vi "main.vi"(8 "error in (no error)":errorcluster, 10 "stages":refnum<class "_stage.lvclass">[](array[class]), 11 "_camera":refnum<class "_camera.lvclass">) -> ()   [LabVIEW 2019]
uses:
  _camera/_camera.lvlibp/_cameraClass/_camera.lvclass
  _stage/_stage.lvlibp/_stageClass/_stage.lvclass
  _dataProcessing/_dataProcessing.lvlibp/_dataProcessingClass/_dataProcessing.lvclass
  <vilib>/Analysis/6fits.llb/Curve Fitting Criteria.ctl
  data_process.ctl
  state.ctl
  <vilib>/Analysis/baseanly.llb/Mean (DBL).vi
  _camera/_camera.lvlibp/_cameraClass/Write stage positions.vi
  _camera/_camera.lvlibp/_cameraClass/Read camera name and version.vi
  _camera/_camera.lvlibp/_cameraClass/Read wavelength.vi
  _camera/_camera.lvlibp/_cameraClass/Write background.vi
  <vilib>/gmath/NumericalOptimization/Nonlinear Curve Fit LM formula string.vi
  _camera/_camera.lvlibp/_cameraClass/Write wavelength.vi
  <vilib>/Utility/file.llb/Read Delimited Spreadsheet (DBL).vi
  <vilib>/Utility/config.llb/Write Key (Double).vi
  <vilib>/Utility/config.llb/Write Key (String).vi
  <vilib>/Utility/config.llb/Read Key (Double).vi
  <vilib>/Utility/config.llb/Read Key (String).vi
  <vilib>/Analysis/NI_AALBase.lvlib
  <vilib>/Utility/Data Type/NI_Data Type.lvlib
  <vilib>/Analysis/NI_AALPro.lvlib
  <vilib>/Utility/config.llb/NI_LVConfig.lvlib
  <vilib>/gmath/NI_Gmath.lvlib
panel:
  in  "is stage reversed?":bool=TRUE
  in  "Experimenter":string="who are you?"
  in  "Title":string="A clever title"
  in  "Experimental parameters (will be saved)":string="sample:\nsolvent:\ncuvette:\noptical density:\nexcitation wavelength:\nexcitation power:\nexcitation spot size:\nexcitation fluence: \nprobe spot size:\ncomment:"
  in  "method":T1 items=["Least Square", "Least Absolute Residual", "Bisquare"]
  out "amplitude":dbl format="%#_3g"
  out "power":dbl format="%#_3g"
  out "offset":dbl format="%#_3g"
  in  "parameter bounds":T2={"amp min"=-inf, "amp max"=inf, "power min"=-inf, "power max"=inf, "offset min"=0.0, "offset max"=600.0}
  out "current scan":i32
  in  "N scans":u16=5
  in  "sample":string="testSample"
  in  "Experiment":string="testExp"
  in  "center cursor":bool=TRUE
  in  "save flag":bool
  in  "save type":bool[](array[boolean])=[FALSE, FALSE, FALSE, FALSE]
  in  "data folder":path=path "Z:/11 Setups/04 NOPA TA/01 Data"
  out "progress":u8(slide) scale=0.0..100.0
  out "scan progress":u8(slide) scale=0.0..100.0
  out "Cursor position (wl)":dbl[](array[numeric])
  out "Cursor position (idx)":dbl[](array[numeric])
  in  "ampl":cluster{dbl, dbl}(slide)={1.567404426559356, 6.9678068410462775} scale=-1.0..10.0
  in  "diff":dbl(slide)=26.28128772635815 scale=0.05..50.0
  out "main graph":cluster{"wavelength":dbl[], "ref mean":dbl[]}[](graph)
  out "Boolean 2":bool
  in  "_dataProcessing.lvlibp:_dataProcessing.lvclass":refnum<class "_dataProcessing.lvclass">
  in  "time delay file":path=path "D:/github/TransientAbsorptionDAQ.lv/stepfiles/01_coarseSteps_-1000_1000fs.txt"
  in  "scan":bool
  in  "bottom panel":u16(ring)=2 items=["x/y", "y/x", "traces", "std", "debug", "parameters", "wavelength"]
  in  "parity?":enum32{"Item 0", "Item 1"}(radio)
  out "Camera initialised?":bool[](array[boolean])
  in  "Algorithm":u16(ring) items=["<(S*-S)/S>/ln(10)", "<S*/S>-1", "<S*/PD*>/<S/PD>", "<S*/Sref*>/<S/Sref>", "<S*/Sref*>/<S/Sref>_alt"]
  out "Char":i16
  in  "view error anal":bool
  in  "view full data":bool
  in  "get bg":bool
  in  "cont acq":bool
  in  "move stage":enum32{"Item 0", "Item 1"}(radio)
  out "timed out?":bool
  out "Boolean":bool
  out "value":dbl
  out "index of element":i32
  out "Stage(s) initialized":bool[](array[boolean])
  out "data processing timing":u32=150
  out "data":variant
  in  "set as t0":bool[](array[boolean])
  in  "home stages":bool[](array[boolean])
  out "stage name(s)":i32[](listbox)
  out "is moving?":bool[](array[boolean]) caption="mov?"
  in  "Listbox":i32(listbox)=1
  out "Tab Control":T3(tab)=enum."wavelength"
  out "Intensity Chart":dbl[][](graph)
  out "Intensity Graph":dbl[][](graph)
  out "Waveform Chart":dbl[](graph)
  out "std graph":cluster{"wavelength":dbl[], "ref std":dbl[]}[](graph)
  out "skipped/missing acqusition":bool
  out "chopper out":bool[][](array[boolean])
  out "synchronization error":bool
  in  "save raw data":bool caption="saw raw data"
  in  "baseline offset (reference)":dbl
  in  "baseline offset (signal)":dbl
  in  "history length":i32=20
  in  "Scale.Range:Maximum":dbl=50.0
  in  "camera max scale":u16(ring) items=["16-bit", "14-bit", "12-bit"]
  in  "save wl calibration to .ini":bool caption="calibrate_wl"
  in  "index":u16
  in  "calibrate wavelength":bool caption="calibrate_wl"
  out "wavelength fit":cluster{i32[], dbl[]}[](graph)
  out "wavelength (fitted)":dbl[](array[numeric]) format="%#.0f"
  in  "wavelength \n(calibration value)":dbl[](array[numeric])=[500.0, 700.0, 550.0, 600.0, 650.0, 450.0, 880.0, 400.0, 800.0] caption="wavelength (calibration value)"
  in  "pixel/index":u16[](array[numeric])=[582, 793, 653, 712, 756, 496, 883, 352, 853]
  in  "mirror?":bool
  in  "initial parameters":dbl[](array[numeric])=[150.0, 200000.0, 1200.0]
  out "best fit parameters":dbl[](array[numeric])
  in  "t0 position(s)":dbl[](array[numeric]) caption="t0 (s)" format="%09.1f"
  out "stage position(s) readback":dbl[](array[numeric]) caption="readback (fs)" format="%09.1f"
  in  "stage position(s)":dbl[](array[numeric]) caption="set (fs)" format="%09.1f"
  out "camera name, version":string
  in  "get_single_acq":bool caption="get single"
  out "vi running?":bool
  out "Processing time":u32(knob)=150 scale=0.0..2000.0
  # "just temp ..."
  # "scan #"
  # "out of"
  # "transient"
  # "pumped mean"
  # "unpumped mean"
  # "reference mean"
  # "Hartmann dispersion formula:"
  # "d(\\lambda) = a1 + a2 / (pix - a3)"
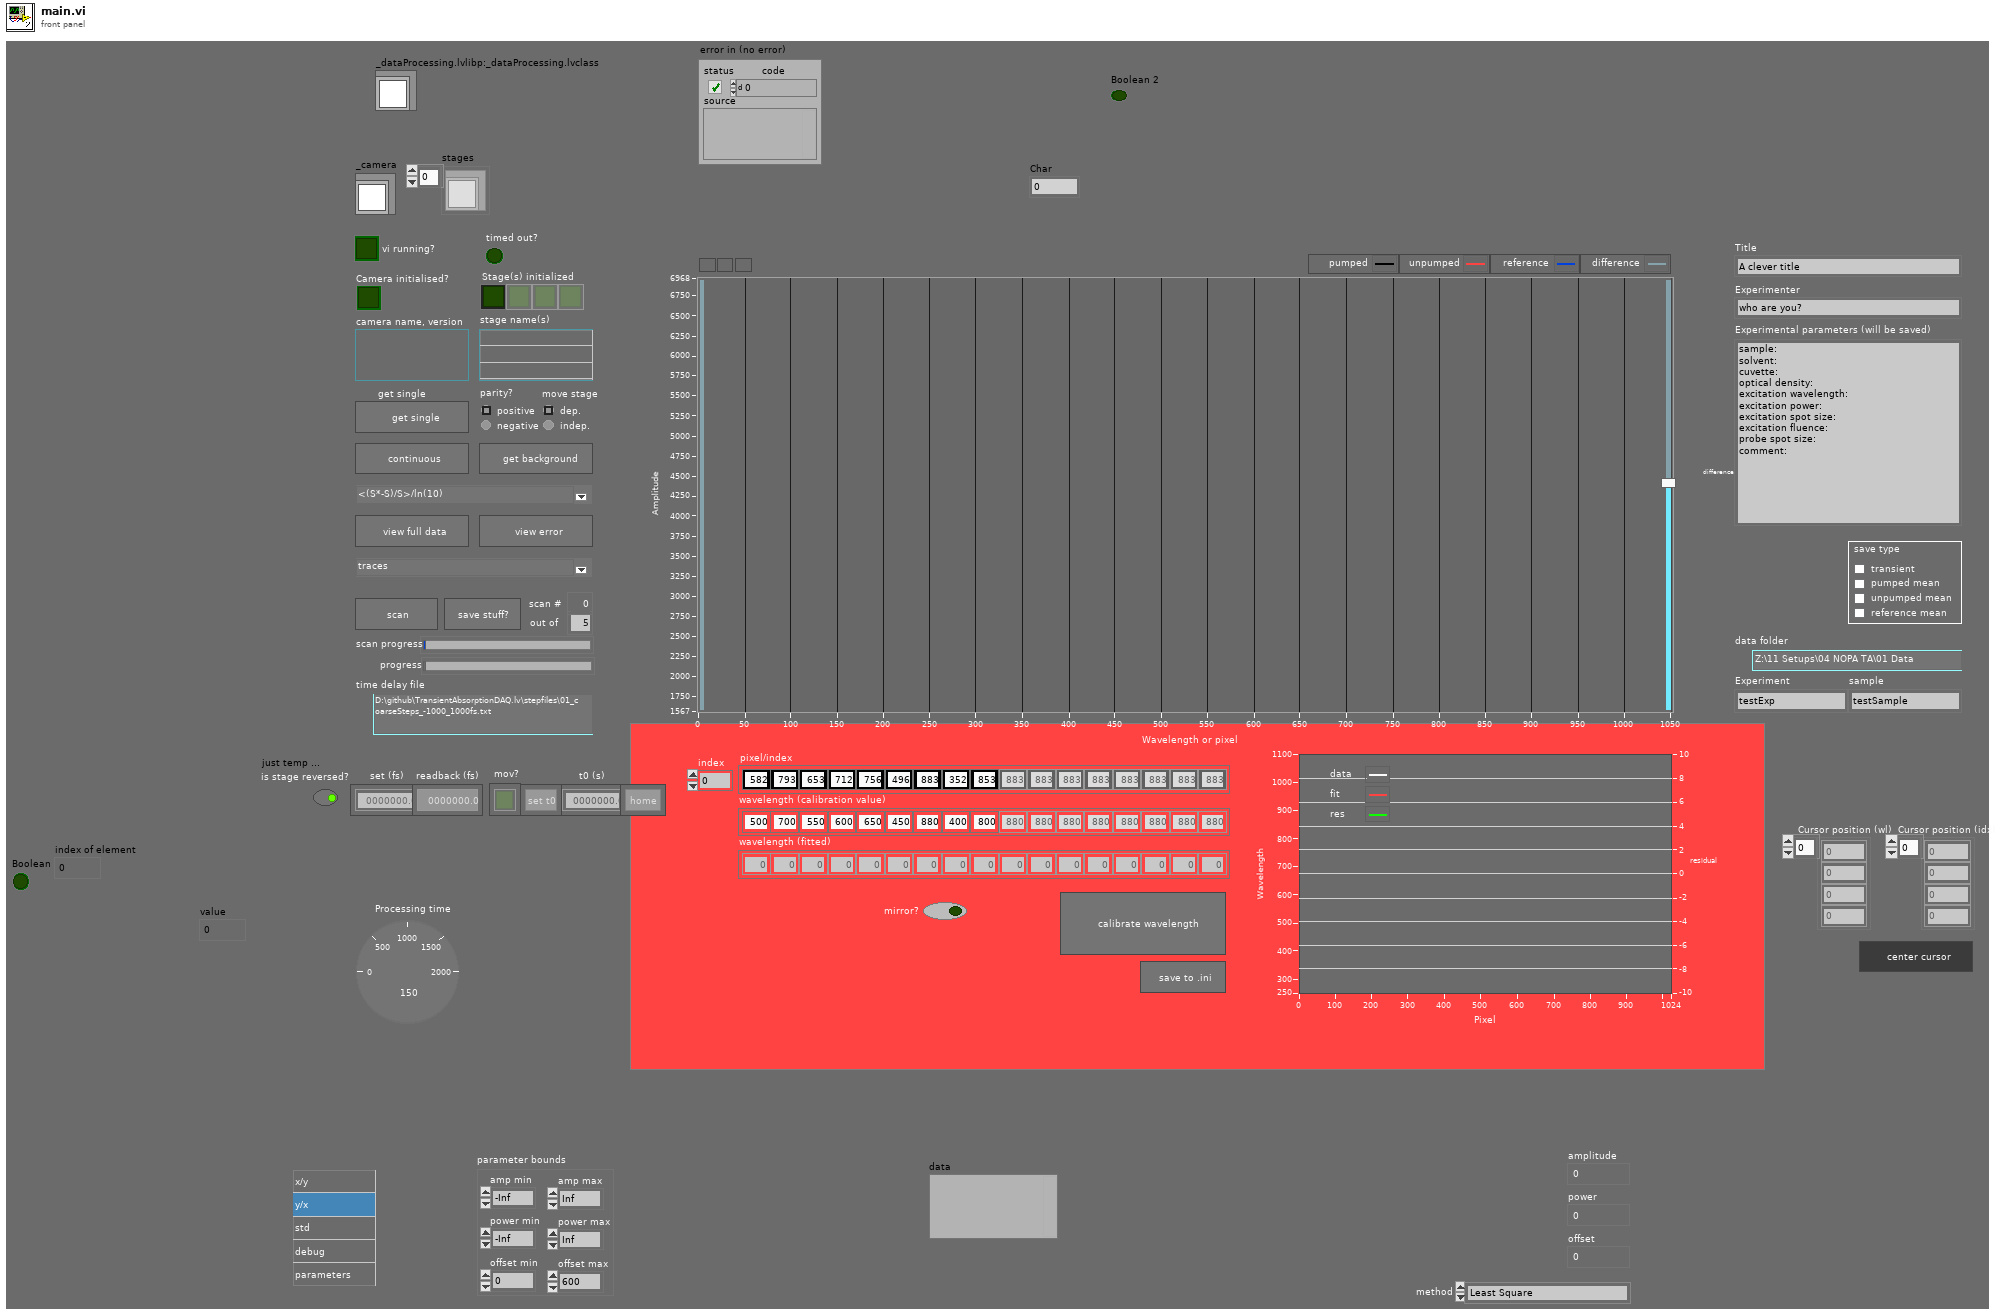
[diagram p1: front panel]
types:
  T1 = typedef "NI_AALPro.lvlib/Curve Fitting Criteria.ctl" = u16
  T2 = cluster{"amp min":dbl, "amp max":dbl, "power min":dbl, "power max":dbl, "offset min":dbl, "offset max":dbl}
  T3 = enum32{"x/y", "y/x", "traces", "std", "debug", "parameters", "wavelength"}
  T4 = typedef "state.ctl" = enum16{"timeout", "hw_init", "sw_init", "cam_single_acq", "cam_get_bg", "cam_rst_bg", "cam_cnt_acq", "cam_set_wl", "stg_set_pos", "stg_home", "scn_load_step_file", "scn_init", "scn_next_step", "scn_next_iter", "dat_update_save_flag", "dat_update_save_type", "dat_save_raw", "dat_send_to_process", "dat_save_wl_to_ini", "stop"}
  T5 = cluster{"acq num":u32[], "transients":dbl[][], "curr acq":i32, "transient":dbl[], "pumped mean":dbl[], "unpumped mean":dbl[], "reference mean":dbl[], "pumped std":dbl[], "unpumped std":dbl[], "reference std":dbl[]}
  T6 = typedef "data_process.ctl" = enum16{"timeout", "init", "reset", "process", "plot", "save", "exit"}
  T7 = cluster{"TA":cluster{"raw data":dbl[][][], "wavelength":dbl[], "trigger":bool[][], "stage position (set) [fs]":dbl[], "stage position (readback) [fs]":dbl[], "scn_step_pos":dbl[], "scn_step_time_dly":dbl[], "scn_step":i32, "scn_iter":i32, "command":T6, "save flag":bool, "save path":path, "save type":bool[]}, "2D":cluster{"wavelength":dbl[]}}
  T8 = enum32{"invalid app kind", "Development System", "Run Time System", "Student Edition", "Embedded LabVIEW", "Evaluation", "Custom"}
  T9 = cluster{"[0]":variant, "[1]":variant, "[2]":variant, "[3]":variant, "[4]":variant, "[5]":variant, "[6]":variant, "[7]":variant, "[8]":variant}
  T10 = typedef "NI_LVConfig.lvlib/Config Data RefNum.ctl" = refnum<k1>
  T11 = cluster{"raw data":dbl[][][], "wavelength":dbl[], "trigger":bool[][], "stage position (set) [fs]":dbl[], "stage position (readback) [fs]":dbl[], "scn_step_pos":dbl[], "scn_step_time_dly":dbl[], "scn_step":i32, "scn_iter":i32, "command":T6, "save flag":bool, "save path":path, "save type":bool[]}
  T12 = typedef "LVRangeTypeDef.ctl" = cluster{"Minimum":dbl, "Maximum":dbl, "Increment":dbl, "Minor Increment":dbl, "Start":dbl}
  T13 = cluster{"wavelength":dbl[], "unpumped mean":dbl[]}
  T14 = cluster{"wavelength":dbl[], "reference mean":dbl[]}
  T15 = typedef "LVCursorListTypeDef.ctl" = cluster{"Name":string, "Color":u32, "Style":u8, "Point Style":u8, "Name Visible":bool, "Allow Drag":bool, "Cursor Mode":u32, "Plot":i32, "Index":i32, "Position":cluster{"X":dbl, "Y":dbl}, "X Scale":u32, "Y Scale":u32, "Watch Plots":i32[], "Watch All Plots":bool, "Plot Area":i32, "Label Offset":cluster{"X":dbl, "Y":dbl}}[]
  T16 = cluster{"wavelength":dbl[], "unpumped std":dbl[]}
  T17 = cluster{"wavelength":dbl[], "reference std":dbl[]}
  T18 = cluster{"wavelength":dbl[], "reference std":dbl[]}[]
  T19 = cluster{"model":string, "Parameters":string[], "x":string}
  T20 = enum16{"open", "replace", "create", "open or create", "replace or create", "replace or create with confirmation"}
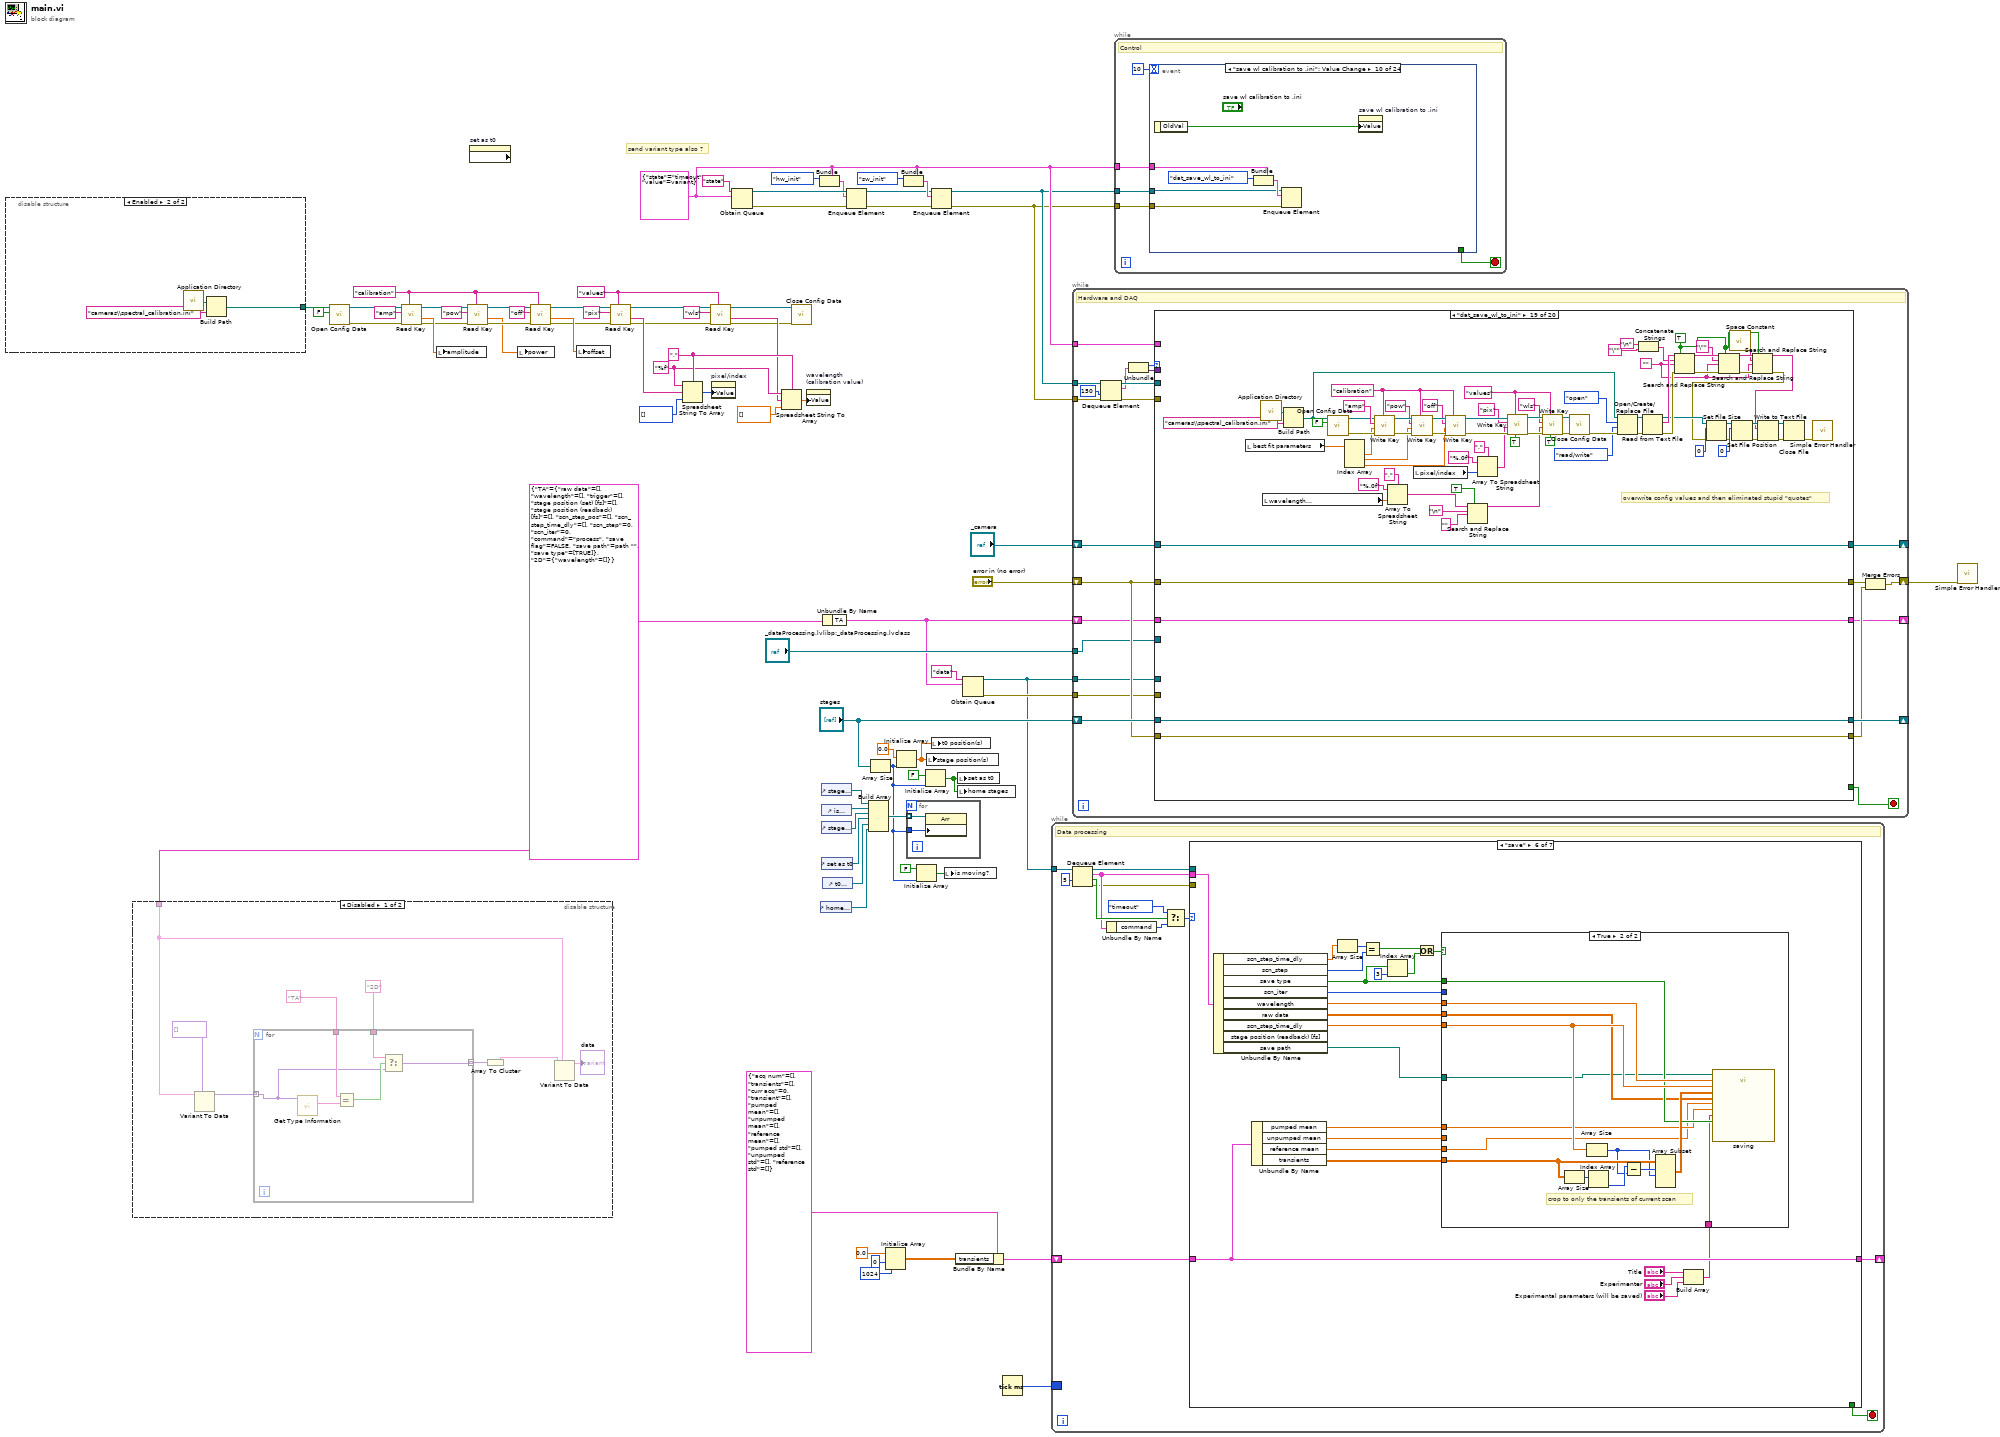
[diagram p0: block diagram]
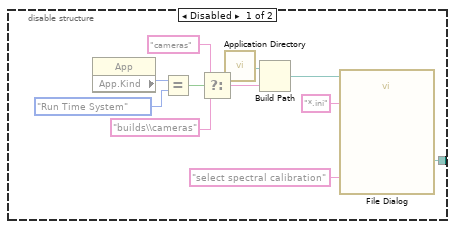
[diagram p2: hidden frame]
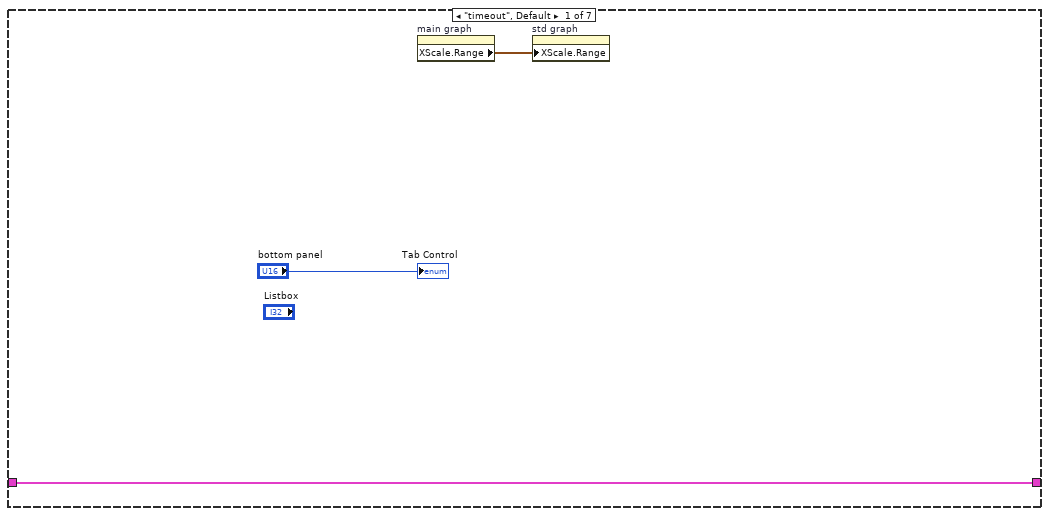
[diagram p4: hidden frame]
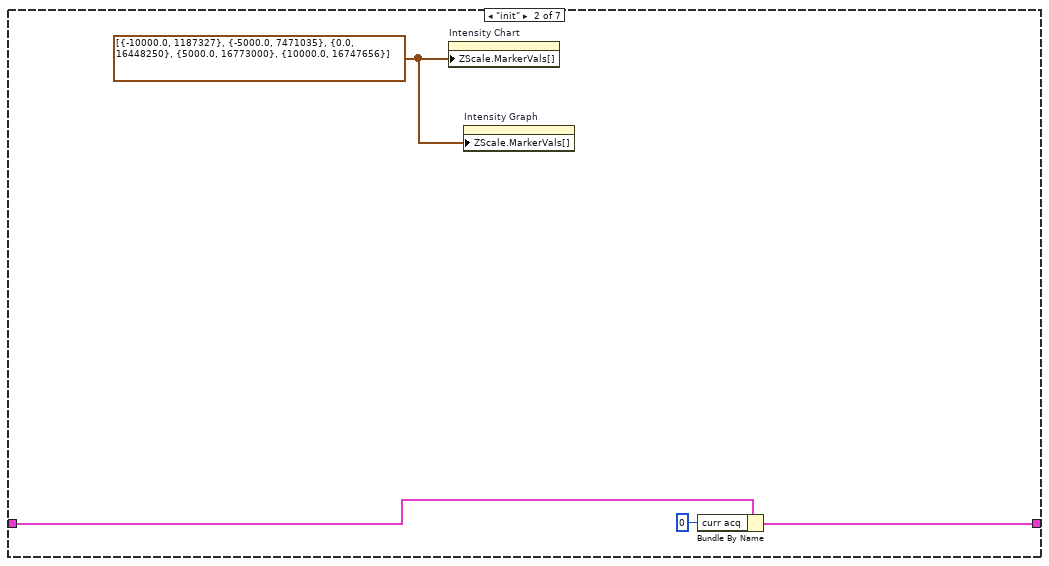
[diagram p5: hidden frame]
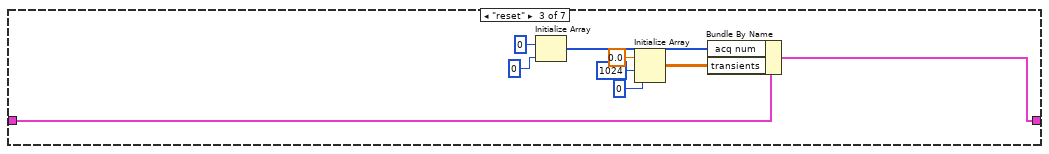
[diagram p6: hidden frame]
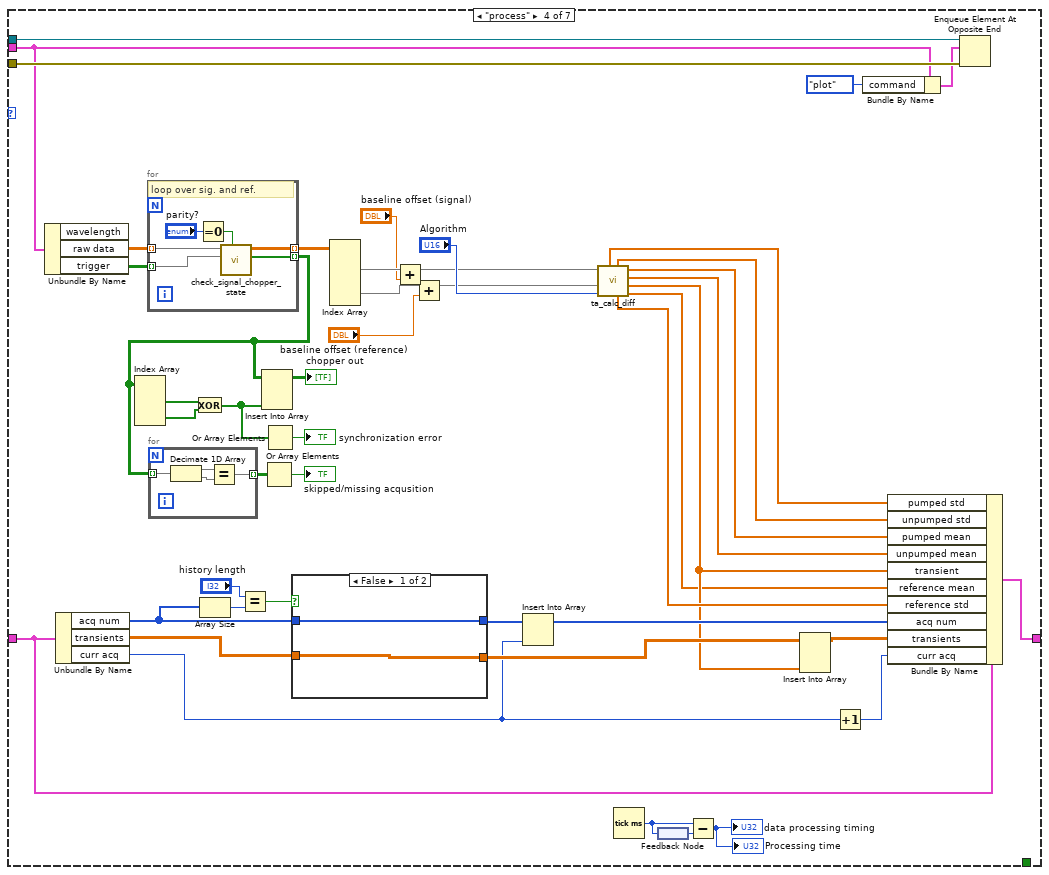
[diagram p7: hidden frame]
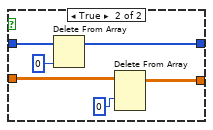
[diagram p8: hidden frame]
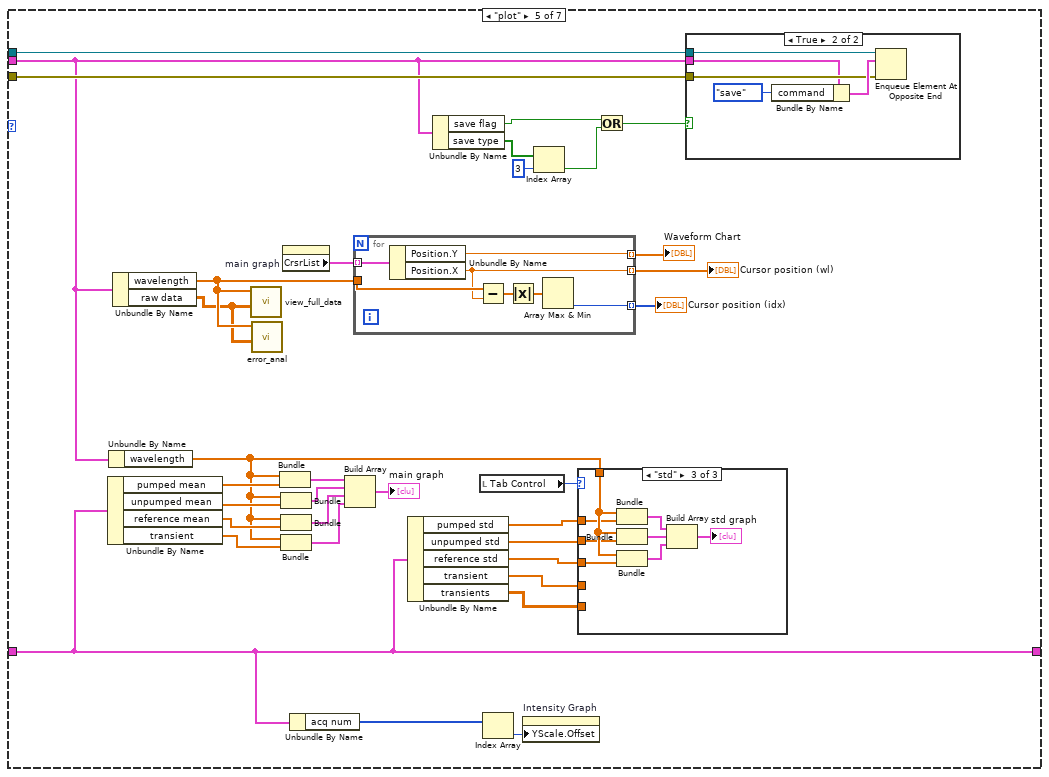
[diagram p9: hidden frame]
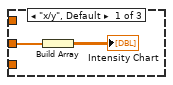
[diagram p11: hidden frame]
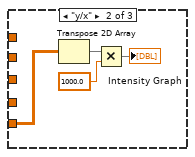
[diagram p12: hidden frame]
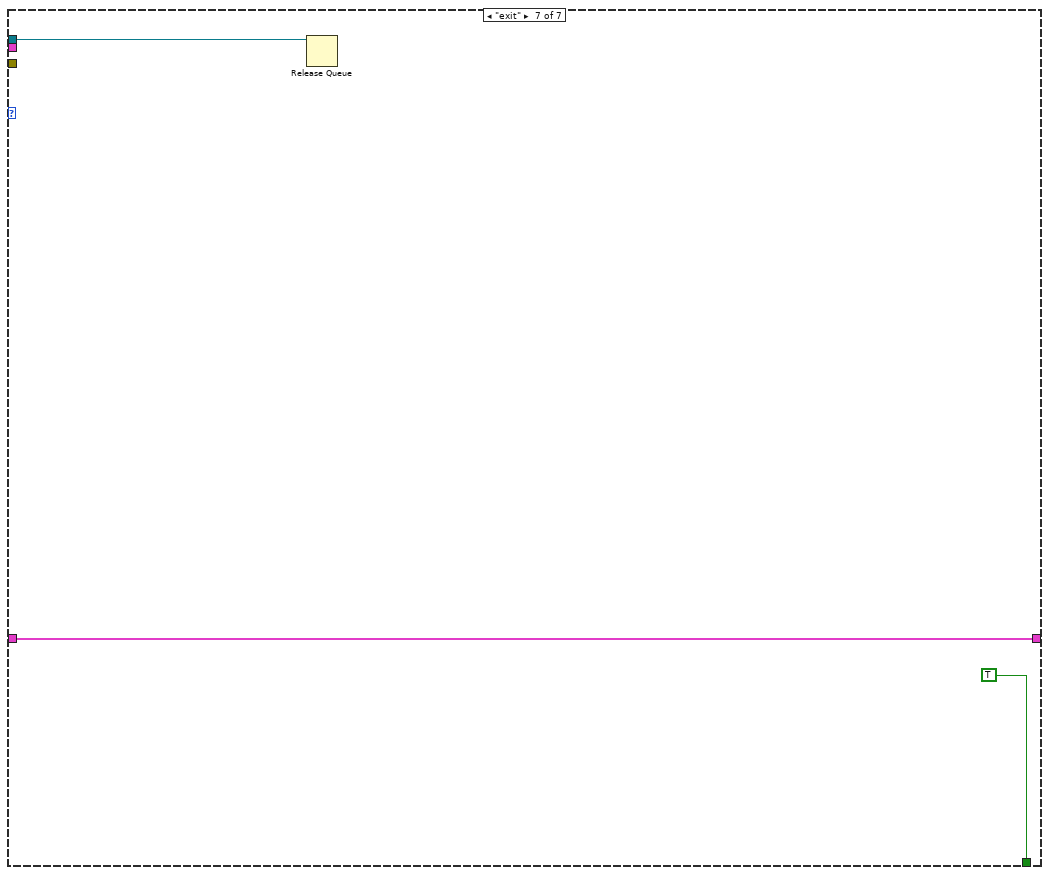
[diagram p14: hidden frame]
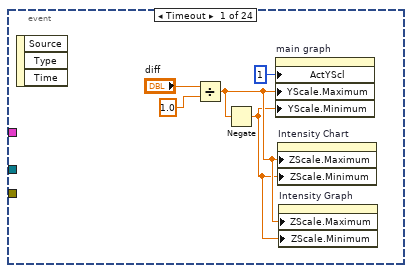
[diagram p15: hidden frame]
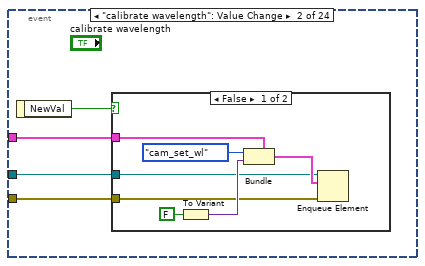
[diagram p16: hidden frame]
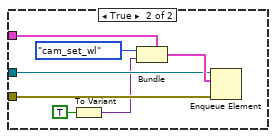
[diagram p17: hidden frame]
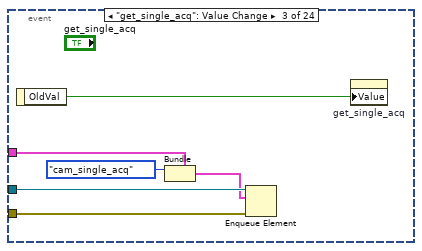
[diagram p18: hidden frame]
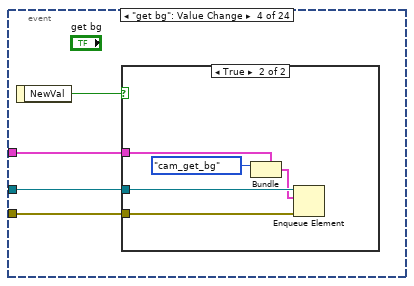
[diagram p19: hidden frame]
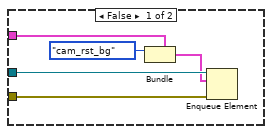
[diagram p20: hidden frame]
diagram:
  w14 = "," ("delimiter (Tab)")
  w13 = "%f" ("format string")
  w15 = "values" ("section")
  w32 = "calibration" ("section")
  w3 = cluster{"state":T4, "value":variant} {"state"=enum."timeout", "value"=variant}
  w42 = T7 {"TA"={"raw data"=[], "wavelength"=[], "trigger"=[], "stage position (set) [fs]"=[], "stage position (readback) [fs]"=[], "scn_step_pos"=[], "scn_step_time_dly"=[], "scn_step"=0, "scn_iter"=0, "command"=enum."process", "save flag"=FALSE, "save path"=path "", "save type"=[TRUE]}, "2D"={"wavelength"=[]}}
  # "send variant type also ?"
  n1 = disable-structure shown="Enabled" {
    disable-tunnel: [w86 w87] -> w38
    frame Disabled {
      n2 = property class="App"() -> ("App.Kind"=w83:T8)  [unwired: 2 in, 2 out]
      n3 = Equal?(x=w83, y=T8."Run Time System") -> (x = y?=w81:bool)
      n4 = Select(t="cameras" ("name or relative path"), s=w81, f="builds\\cameras" ("name or relative path")) -> (s? t:f=w78:string)
      n5 = call <vilib>:"Application Directory.vi"() -> ("Application Directory"=w85:path)
      n6 = Build Path(base path=w85, name or relative path=w78) -> (appended path=w84:path)
      n7 = call "File Dialog"("start path"=w84, "prompt"="select spectral calibration", "pattern (all files)"="*.ini") -> ("selected path"=w86:path)  [unwired: 9 in, 3 out]
    }
    frame Enabled {
      n8 = call <vilib>:"Application Directory.vi"() -> ("Application Directory"=w89:path)
      n9 = Build Path(base path=w89, name or relative path="cameras\\spectral_calibration.ini") -> (appended path=w87:path)
    }
  }
  n10 = disable-structure shown="Disabled" {
    disable-tunnel: w42 -> [w90 _]
    frame Disabled {
      n11 = Variant To Data(type=variant[] [], Variant=w90) -> (data=w96:variant[])  [unwired: 1 in, 1 out]
      n12 = for {
        tunnel: w96 -> [w100] mode=indexing
        tunnel: "TA" ("x") -> [w102]
        tunnel: "2D" -> [w99]
        tunnel: [w98] -> w93 mode=indexing
        n13 = call <vilib>:"Get Type Information.vi"("variant"=w100) -> ("name"=w103:string)  [unwired: 6 in, 4 out]
        n14 = Equal?(x=w102, y=w103) -> (x = y?=w101:bool)
        n15 = Select(t=w99, s=w101, f=w100) -> (s? t:f=w98:variant)
      }
      n16 = Array To Cluster(array=w93) -> (cluster=w92:T9)
      n17 = Variant To Data(type=w90, Variant=w92) -> (data=→"data":T7)  [unwired: 1 in, 1 out]
    }
    frame Enabled {
    }
  }
  n18 = call <vilib>:"Open Config Data.vi"("create file if necessary (T)"=FALSE, "configuration file path"=w38) -> ("error out"=w36:errorcluster, "refnum"=w37:T10)  [unwired: 7 in, 1 out]
  n19 = call-poly <vilib>:"Read Key.vi"("section"=w32, "error in (no error)"=w36, "key"="amp", "refnum"=w37) -> ("error out"=w29:errorcluster, "value"=w31:dbl, "refnum out"=w30:T10)  [unwired: 4 in, 1 out]
  n20 = local write "amplitude"(w31) -> ()
  n21 = call-poly <vilib>:"Read Key.vi"("section"=w32, "error in (no error)"=w29, "key"="pow", "refnum"=w30) -> ("error out"=w28:errorcluster, "value"=w26:dbl, "refnum out"=w27:T10)  [unwired: 4 in, 1 out]
  n22 = property on="set as t0" class="Arr" props=["Number of Rows"]() -> ()  [unwired: 2 in, 3 out]
  n23 = local write "power"(w26) -> ()
  n24 = call-poly <vilib>:"Read Key.vi"("section"=w32, "error in (no error)"=w28, "key"="off", "refnum"=w27) -> ("error out"=w23:errorcluster, "value"=w25:dbl, "refnum out"=w24:T10)  [unwired: 4 in, 1 out]
  n25 = local write "offset"(w25) -> ()
  n26 = call-poly <vilib>:"Read Key.vi"("section"=w15, "error in (no error)"=w23, "key"="pix", "refnum"=w24) -> ("error out"=w16:errorcluster, "value"=w22:string, "refnum out"=w17:T10)  [unwired: 4 in, 1 out]
  n27 = Spreadsheet String To Array(delimiter (Tab)=w14, format string=w13, spreadsheet string=w22, array type (2D Dbl)=i32[] []) -> (array=w19:i32[])
  n28 = call-poly <vilib>:"Read Key.vi"("section"=w15, "error in (no error)"=w16, "key"="wls", "refnum"=w17) -> ("error out"=w8:errorcluster, "value"=w12:string, "refnum out"=w9:T10)  [unwired: 4 in, 1 out]
  n29 = property on="pixel/index" class="Arr (strict)"("Value"=w19) -> ()  [unwired: 2 in, 2 out]
  n30 = Obtain Queue(name (unnamed)="state", element data type=w3) -> (queue out=w73:refnum<queue>, error out=w72:errorcluster)  [unwired: 3 in, 1 out]
  n31 = Spreadsheet String To Array(delimiter (Tab)=w14, format string=w13, spreadsheet string=w12, array type (2D Dbl)=dbl[] []) -> (array=w10:dbl[])
  n32 = call <vilib>:"Close Config Data.vi"("error in (no error)"=w8, "refnum"=w9) -> ()  [unwired: 8 in, 2 out]
  n33 = property on="wavelength \n(calibration value)" class="Arr (strict)"("Value"=w10) -> ()  [unwired: 2 in, 2 out]
  n34 = Bundle(cluster=w3, "state"=state."hw_init") -> (w59:cluster{"state":T4, "value":variant})  [unwired: 1 in]
  n35 = control-ref of="home stages"() -> (w60:refnum<vi>)
  n36 = control-ref of="stage position(s)"() -> (w63:refnum<vi>)
  n37 = control-ref of="is moving?"() -> (w66:refnum<vi>)
  n38 = control-ref of="stage position(s) readback"() -> (w65:refnum<vi>)
  n39 = control-ref of="set as t0"() -> (w62:refnum<vi>)
  n40 = Unbundle By Name(w42) -> ("TA"=w41:T11)
  n41 = control-ref of="t0 position(s)"() -> (w61:refnum<vi>)
  n42 = Enqueue Element(queue=w73, element=w59, error in (no error)=w72) -> (queue out=w5:refnum<queue>, error out=w4:errorcluster)  [unwired: 1 in, 1 out]
  n43 = Build Array(w63, w66, w65, w62, w61, w60) -> (w64:refnum<vi>[])
  n44 = Array Size(array="stages") -> (size(s)=w55:i32)
  n45 = Initialize Array(0.0, 0 ("dimension size"), 1024 ("dimension size")) -> (w47:dbl[][])
  n46 = Initialize Array(0.0, w55) -> (w54:dbl[])
  n47 = Bundle(cluster=w3, "state"=state."sw_init") -> (w7:cluster{"state":T4, "value":variant})  [unwired: 1 in]
  n48 = for {
    tunnel: w64 -> [w104] mode=indexing
    tunnel: w55 -> [w105]
    n49 = property class="Arr"(reference=w104, "Number of Rows"=w105) -> ()  [unwired: 1 in, 2 out]
  }
  n50 = Initialize Array(FALSE, w55) -> (w58:bool[])
  n51 = Initialize Array(FALSE, w55) -> (w53:bool[])
  n52 = local write "stage position(s)"(w54) -> ()
  n53 = Enqueue Element(queue=w5, element=w7, error in (no error)=w4) -> (queue out=w2:refnum<queue>, error out=w1:errorcluster)  [unwired: 1 in, 1 out]
  n54 = local write "t0 position(s)"(w54) -> ()
  n55 = local write "is moving?"(w58) -> ()
  n56 = Bundle By Name(cluster=T5 {"acq num"=[], "transients"=[], "curr acq"=0, "transient"=[], "pumped mean"=[], "unpumped mean"=[], "reference mean"=[], "pumped std"=[], "unpumped std"=[], "reference std"=[]}, "transients"=w47) -> (w48:T5)
  n57 = local write "set as t0"(w53) -> ()
  n58 = local write "home stages"(w53) -> ()
  n59 = Obtain Queue(name (unnamed)="data", element data type=w41) -> (queue out=w40:refnum<queue>, error out=w43:errorcluster)  [unwired: 3 in, 1 out]
  n60 = Tick Count (ms)() -> (millisecond timer value=w67:u32)
  n61 = while {
    border: w67 -> [_]
    shift-right: [w113] -> _
    shift-left: w48 -> [w114]
    tunnel: w40 -> [w112]
    stop <- w117 stop-if-true
    # "Data processing"
    n62 = Dequeue Element(queue=w112, timeout in ms (-1)=5) -> (queue out=w109:refnum<queue>, element=w108:T11, timed out?=w110:bool, error out=w107:errorcluster)  [unwired: 1 in]
    n63 = Unbundle By Name(w108) -> ("command"=w106:T6)
    n64 = Select(t=data_process."timeout", s=w110, f=w106) -> (s? t:f=w115:T6)
    n65 = case shown="\"save\"" w115 {
      tunnel: [_ _ _ _ _ _ TRUE] -> w117
      tunnel: w114 -> [w120 w123 w128 w157 w214 w277 w295]
      tunnel: [w120 w121 w125 w158 w214 w277 w295] -> w113
      tunnel: w109 -> [_ _ _ w152 w205 _ w294]
      tunnel: w108 -> [_ _ _ w146 w203 w279 _]
      tunnel: w107 -> [_ _ _ w151 w204 _ _]
      frame "timeout", Default {
        n66 = property on="main graph" class="XYGraph (strict)"() -> ("XScale.Range"=w118:T12)  [unwired: 2 in, 2 out]
        n67 = property on="std graph" class="XYGraph (strict)"("XScale.Range"=w118) -> ()  [unwired: 2 in, 2 out]
        "Tab Control" <- "bottom panel"
      }
      frame "init" {
        w124 = cluster{dbl, u32}[] [{-10000.0, 1187327}, {-5000.0, 7471035}, {0.0, 16448250}, {5000.0, 16773000}, {10000.0, 16747656}] ("Z Scale.Marker Values[]")
        n68 = property on="Intensity Chart" class="IntChart (strict)"("ZScale.MarkerVals[]"=w124) -> ()  [unwired: 2 in, 2 out]
        n69 = property on="Intensity Graph" class="IntGraph (strict)"("ZScale.MarkerVals[]"=w124) -> ()  [unwired: 2 in, 2 out]
        n70 = Bundle By Name(cluster=w123, "curr acq"=0) -> (w121:T5)
      }
      frame "reset" {
        n71 = Initialize Array(u32 0 ("element"), 0 ("dimension size")) -> (w127:u32[])
        n72 = Initialize Array(0.0 ("element"), 1024 ("dimension size"), 0 ("dimension size")) -> (w126:dbl[][])
        n73 = Bundle By Name(cluster=w128, "acq num"=w127, "transients"=w126) -> (w125:T5)
      }
      frame "process" {
        n74 = Unbundle By Name(w146) -> ("raw data"=w179:dbl[][][], "trigger"=w178:bool[][])  [unwired: 1 out]
        n75 = Unbundle By Name(w157) -> ("acq num"=w162:u32[], "transients"=w161:dbl[][], "curr acq"=w156:i32)
        n76 = for {
          tunnel: w179 -> [w197] mode=indexing
          tunnel: w178 -> [w195] mode=indexing
          tunnel: [w196] -> w177 mode=indexing
          tunnel: [w194] -> w155 mode=indexing
          # "loop over sig. and ref."
          n77 = Equal To 0?(x="parity?") -> (x = 0?=w193:bool)
          n78 = call "check_signal_chopper_state.vi"("parity?"=w193, "chopper"=w195, "data"=w197) -> ("chopper out"=w194:bool[], "data out"=w196:dbl[][])  [unwired: 7 in]
        }
        n79 = Index Array(array=w155) -> (element #1=w174:bool[], element #2=w173:bool[])  [unwired: 4 in]
        n80 = for {
          tunnel: w155 -> [w183] mode=indexing
          tunnel: [w180] -> w154 mode=indexing
          n81 = Decimate 1D Array(w183) -> (w182:bool[], w181:bool[])
          n82 = Equal?(x=w182, y=w181) -> (x = y?=w180:bool[])
        }
        n83 = Exclusive Or(1:w173, 2:w174) -> (0:w168:bool[])
        n84 = Array Size(array=w162) -> (size(s)=w164:i32)
        n85 = Equal?(x="history length", y=w164) -> (x = y?=w163:bool)
        n86 = Insert Into Array(array=w155, new element=w168) -> (→"chopper out":bool[][])  [unwired: 2 in]
        n87 = Or Array Elements(Boolean array=w154) -> (logical OR=→"skipped/missing acqusition":bool)
        n88 = Or Array Elements(Boolean array=w168) -> (logical OR=→"synchronization error":bool)
        n89 = case shown="False" w163 {
          tunnel: w162 -> [w185 w191]
          tunnel: [w185 w189] -> w159
          tunnel: w161 -> [w184 w188]
          tunnel: [w184 w187] -> w160
          frame False {
          }
          frame True {
            n90 = Delete From Array(array=w191, index=0) -> (array with subset deleted=w189:u32[])  [unwired: 1 in, 1 out]
            n91 = Delete From Array(array=w188, index (row)=0 ("disabled index (col)")) -> (array with subset deleted=w187:dbl[][])  [unwired: 2 in, 1 out]
          }
        }
        n92 = Index Array(array=w177) -> (element #1=w176:dbl[][], element #2=w175:dbl[][])  [unwired: 6 in]
        n93 = Add(x=w176, y="baseline offset (signal)") -> (x+y=w150:dbl[][])
        n94 = Add(x=w175, y="baseline offset (reference)") -> (x+y=w149:dbl[][])
        n95 = Insert Into Array(array=w159, new element=w156) -> (w137:u32[])  [unwired: 1 in]
        n96 = call "ta_calc_diff.vi"("Algorithm"="Algorithm", "ref in"=w149, "data in"=w150) -> ("ref mean"=w134:dbl[], "diff"=w135:dbl[], "unpumped"=w142:dbl[], "pumped"=w143:dbl[], "ref std"=w136:dbl[], "unpumped std"=w141:dbl[], "pumped std"=w140:dbl[])  [unwired: 2 in]
        n97 = Tick Count (ms)() -> (millisecond timer value=w171:u32)
        n98 = feedback #1() -> (w170:u32)
        n99 = feedback-in #1(w171) -> ()
        n100 = Subtract(x=w171, y=w170) -> (x-y=→"data processing timing" →"Processing time":u32)
        n101 = Insert Into Array(array=w160, new element=w135) -> (w138:dbl[][])  [unwired: 2 in]
        n102 = Increment(x=w156) -> (x+1=w139:i32)
        n103 = Bundle By Name(cluster=w146, "command"=data_process."plot") -> (w145:T11)
        n104 = Bundle By Name(cluster=w157, "pumped std"=w140, "unpumped std"=w141, "pumped mean"=w143, "unpumped mean"=w142, "transient"=w135, "reference mean"=w134, "reference std"=w136, "acq num"=w137, "transients"=w138, "curr acq"=w139) -> (w158:T5)
        n105 = Enqueue Element At Opposite End(queue=w152, element=w145, error in (no error)=w151) -> ()  [unwired: 1 in, 3 out]
      }
      frame "plot" {
        n106 = Unbundle By Name(w214) -> ("pumped mean"=w226:dbl[], "unpumped mean"=w225:dbl[], "reference mean"=w224:dbl[], "transient"=w223:dbl[])
        n107 = Unbundle By Name(w203) -> ("wavelength"=w220:dbl[])
        n108 = Unbundle By Name(w203) -> ("wavelength"=w207:dbl[], "raw data"=w206:dbl[][][])
        n109 = call "view_full_data.vi"("data"=w206, "wavelength"=w207) -> ()  [unwired: 10 in]
        n110 = call "error_anal.vi"("data"=w206, "wavelength"=w207) -> ()  [unwired: 10 in]
        n111 = Bundle("wavelength"=w220, "pumped mean"=w226) -> (w230:cluster{"wavelength":dbl[], "pumped mean":dbl[]})  [unwired: 1 in]
        n112 = Bundle("wavelength"=w220, "unpumped mean"=w225) -> (w229:T13)  [unwired: 1 in]
        n113 = Bundle("wavelength"=w220, "reference mean"=w224) -> (w222:T14)  [unwired: 1 in]
        n114 = Bundle("wavelength"=w220, "transient"=w223) -> (w221:cluster{"wavelength":dbl[], "transient":dbl[]})  [unwired: 1 in]
        n115 = property on="main graph" class="XYGraph (strict)"() -> ("CrsrList"=w211:T15)  [unwired: 2 in, 2 out]
        n116 = Unbundle By Name(w214) -> ("acq num"=w213:u32[])
        n117 = Build Array(w230, w229, w222, w221) -> (→"main graph":cluster{"wavelength":dbl[], "transient":dbl[]}[])
        n118 = for {
          tunnel: w211 -> [w242] mode=indexing
          tunnel: w207 -> [w241]
          tunnel: [w240] -> w208 mode=indexing
          tunnel: [w237] -> w210 mode=indexing
          tunnel: [w236] -> w209 mode=indexing
          n119 = Unbundle By Name(w242) -> ("Position.Y"=w240:dbl, "Position.X"=w236:dbl)
          n120 = Subtract(x=w241, y=w236) -> (x-y=w239:dbl[])
          n121 = Absolute Value(x=w239) -> (abs(x)=w238:dbl[])
          n122 = Array Max & Min(array=w238) -> (min index (indices)=w237:i32)  [unwired: 3 out]
        }
        "Cursor position (idx)" <- w210
        "Waveform Chart" <- w208
        "Cursor position (wl)" <- w209
        n123 = Unbundle By Name(w214) -> ("pumped std"=w219:dbl[], "unpumped std"=w218:dbl[], "reference std"=w217:dbl[], "transient"=w216:dbl[], "transients"=w215:dbl[][])
        n124 = Unbundle By Name(w203) -> ("save flag"=w200:bool, "save type"=w202:bool[])
        n125 = local read "Tab Control"() -> (w228:T3)
        n126 = Index Array(array=w213) -> (element=w212:u32)  [unwired: 1 in]
        n127 = property on="Intensity Graph" class="IntGraph (strict)"("YScale.Offset"=w212) -> ()  [unwired: 2 in, 2 out]
        n128 = Index Array(array=w202, index=3) -> (element=w199:bool)
        n129 = case shown="\"std\"" w228 {
          tunnel: w220 -> [_ _ w253]
          tunnel: w219 -> [_ _ w252]
          tunnel: w218 -> [_ _ w251]
          tunnel: w217 -> [_ _ w250]
          tunnel: w216 -> [w243 _ _]
          tunnel: w215 -> [_ w245 _]
          frame "x/y", Default {
            n130 = Build Array(w243) -> (→"Intensity Chart":dbl[][])
          }
          frame "y/x" {
            n131 = Transpose 2D Array(2D array=w245) -> (transposed array=w248:dbl[][])
            n132 = Multiply(x=w248, y=1000.0) -> (x*y=→"Intensity Graph":dbl[][])
          }
          frame "std" {
            n133 = Bundle("wavelength"=w253, "pumped std"=w252) -> (w254:cluster{"wavelength":dbl[], "pumped std":dbl[]})  [unwired: 1 in]
            n134 = Bundle("wavelength"=w253, "unpumped std"=w251) -> (w255:T16)  [unwired: 1 in]
            n135 = Bundle("wavelength"=w253, "reference std"=w250) -> (w256:T17)  [unwired: 1 in]
            n136 = Build Array(w254, w255, w256) -> (→"std graph":T18)
          }
        }
        n137 = Or(x=w200, y=w199) -> (x .or. y?=w198:bool)
        n138 = case shown="True" w198 {
          tunnel: w205 -> [_ w233]
          tunnel: w204 -> [_ w232]
          tunnel: w203 -> [_ w231]
          frame False {
          }
          frame True {
            n139 = Bundle By Name(cluster=w231, "command"=data_process."save") -> (w235:T11)
            n140 = Enqueue Element At Opposite End(queue=w233, element=w235, error in (no error)=w232) -> ()  [unwired: 1 in, 3 out]
          }
        }
      }
      frame "save" {
        n141 = Unbundle By Name(w279) -> ("scn_step_time_dly"=w267:dbl[], "scn_step"=w271:i32, "save type"=w264:bool[], "scn_iter"=w272:i32, "wavelength"=w278:dbl[], "raw data"=w273:dbl[][][], "scn_step_time_dly"=w266:dbl[], "save path"=w268:path)  [unwired: 1 out]
        n142 = Unbundle By Name(w277) -> ("pumped mean"=w276:dbl[], "unpumped mean"=w275:dbl[], "reference mean"=w274:dbl[], "transients"=w269:dbl[][])
        n143 = Array Size(array=w267) -> (size(s)=w270:i32)
        n144 = Equal?(x=w270, y=w271) -> (x = y?=w265:bool)
        n145 = Index Array(array=w264, index=3) -> (element=w263:bool)
        n146 = Or(x=w265, y=w263) -> (x .or. y?=w261:bool)
        n147 = Build Array("Title", "Experimenter", "Experimental parameters (will be saved)") -> (w257:string[])
        n148 = case shown="True" w261 {
          tunnel: w278 -> [_ w293]
          tunnel: w276 -> [_ w283]
          tunnel: w275 -> [_ _]
          tunnel: w274 -> [_ w282]
          tunnel: w273 -> [_ w284]
          tunnel: w264 -> [_ w285]
          tunnel: w272 -> [_ _]
          tunnel: w269 -> [_ w292]
          tunnel: w268 -> [_ w281]
          tunnel: w266 -> [_ w291]
          tunnel: w257 -> [_ w280]
          frame False {
          }
          frame True {
            # "crop to only the transients of current scan"
            n149 = Array Size(array=w292) -> (size(s)=w290:i32[])
            n150 = Array Size(array=w291) -> (size(s)=w287:i32)
            n151 = Index Array(array=w290) -> (element=w289:i32)  [unwired: 1 in]
            n152 = Subtract(x=w289, y=w287) -> (x-y=w288:i32)
            n153 = Array Subset(array=w292, index (row)=w288, length (row)=w287) -> (w286:dbl[][])  [unwired: 2 in]
            n154 = call "saving.vi"("file path (use dialog)"=w281, "save type"=w285, "details"=w280, "signal mean"=w283, "wavelength"=w293, "time delays"=w291, "transients"=w286, "raw data"=w284, "reference mean"=w282) -> ()  [unwired: 7 in]
          }
        }
      }
      frame "exit" {
        n155 = Release Queue(queue=w294) -> ()  [unwired: 2 in, 3 out]
      }
    }
  }
  n156 = while {
    shift-right: [w318] -> _
    shift-left: "_camera" -> [w319]
    tunnel: w2 -> [w301]
    tunnel: w1 -> [w317]
    shift-right: [w309] -> w71
    shift-left: "error in (no error)" -> [w311]
    shift-right: [w313] -> _
    shift-left: "stages" -> [w312]
    tunnel: w3 -> [w303]
    shift-right: [w300] -> _
    shift-left: w41 -> [w307]
    tunnel: "_dataProcessing.lvlibp:_dataProcessing.lvclass" -> [w299]
    tunnel: w40 -> [w298]
    tunnel: w43 -> [w297]
    stop <- w316 stop-if-true
    # "Hardware and DAQ"
    n157 = Dequeue Element(queue=w301, timeout in ms (-1)=150, error in (no error)=w317) -> (queue out=w315:refnum<queue>, element=w305:cluster{"state":T4, "value":variant}, error out=w314:errorcluster)  [unwired: 1 out]
    n158 = Unbundle(w305) -> ("state"=w304:T4, "value"=w302:variant)
    n159 = case shown="\"dat_save_wl_to_ini\"" w304 {
      tunnel: w319 -> [w327 w422 w482 w500 w553 w566 w581 w607 w681 w691 w702 w732 w765 w812 w848 w862 w879 w905 w983 w1007]
      tunnel: [w326 w435 w482 w497 w551 w565 w581 w612 w680 w691 w702 w732 w765 w812 w848 w862 w879 w905 w983 w1006] -> w318
      tunnel: [_ _ _ _ _ _ _ _ _ _ _ _ _ _ _ _ _ _ _ w1008] -> w316
      tunnel: w315 -> [w333 w403 w475 w489 _ _ w585 _ _ _ _ w727 w761 w815 _ _ w892 _ _ w995]
      tunnel: w314 -> [w332 w404 w474 w490 _ _ w584 _ _ _ _ w726 w760 w814 _ _ w891 _ _ w994]
      tunnel: w311 -> [w335 w421 w481 w499 w548 w563 w580 w606 w682 w690 w701 w731 w764 w811 w849 w861 w878 w904 w981 w1004]
      tunnel: [w334 w433 w481 w496 w546 w562 w580 w611 w682 w690 w701 w731 w764 w811 w849 w861 w878 w904 w981 w1002] -> w310
      tunnel: [w328 w414 w479 w492 w545 w561 w579 w610 w674 w689 w700 w730 w762 w810 w851 w856 w875 w903 w979 w998] -> w313
      tunnel: w312 -> [w331 w431 w479 w495 w545 w561 w579 w610 w677 w689 w700 w730 w762 w810 w851 w856 w875 w903 w979 w1001]
      tunnel: w311 -> [w330 w428 w478 w494 w544 w560 w578 w609 w679 w688 w699 w729 w763 w809 w850 w855 w874 w902 w980 w1000]
      tunnel: [w329 w413 w478 w493 w544 w560 w578 w609 w671 w688 w699 w729 w763 w809 w850 w855 w874 w902 w980 w999] -> w308
      tunnel: w307 -> [w320 w429 w480 w498 w543 w559 w568 w608 w666 w687 w694 w724 w758 w808 w853 w860 w873 w895 w982 w1003]
      tunnel: w303 -> [w325 w405 w473 w488 _ _ w571 _ _ _ _ w725 w759 w813 _ _ w882 _ _ w989]
      tunnel: w302 -> [w324 _ _ _ _ _ _ w598 w670 _ w698 _ _ _ w847 w857 _ w901 _ _]
      tunnel: [w320 w408 w480 w483 w543 w559 w568 w608 w666 w687 w693 w722 w757 w816 w852 w859 w872 w895 w982 w985] -> w300
      tunnel: w299 -> [_ w402 _ _ _ _ _ _ _ _ _ _ _ _ _ _ _ _ _ _]
      tunnel: w298 -> [_ _ _ _ _ _ _ _ _ _ _ _ _ _ _ _ _ w897 _ w987]
      tunnel: w297 -> [_ _ _ _ _ _ _ _ _ _ _ _ _ _ _ _ _ w896 _ w986]
      frame "timeout", Default {
        w322 = TRUE ("Boolean 2")
        n160 = case shown="No Error" w335 {
          selector: w335 -> [w347 w398]
          tunnel: [w348 w398] -> w334
          tunnel: w333 -> [_ w400]
          tunnel: w332 -> [_ w399]
          tunnel: w331 -> [w344 w396]
          tunnel: w330 -> [w346 w395]
          tunnel: [w345 w395] -> w329
          tunnel: [w343 w396] -> w328
          tunnel: w327 -> [w350 w397]
          tunnel: [w349 w397] -> w326
          tunnel: w325 -> [_ w394]
          tunnel: w324 -> [_ _]
          tunnel: [FALSE TRUE ("Boolean")] -> w323
          tunnel: w322 -> [w340 w388]
          tunnel: [w339 w387] -> w321
          frame No Error {
            n161 = First Call?() -> (First Call?: T/F=w337:bool)
            n162 = case shown="True" w337 {
              tunnel: w346 -> [w356 w372]
              tunnel: [w355 w370] -> w345
              tunnel: w344 -> [w354 w373]
              tunnel: [w353 w371] -> w343
              tunnel: [w352 w369] -> w341
              tunnel: [w351 w368] -> w336
              frame False {
                n163 = for {
                  shift-right: [w357] -> w355
                  shift-left: w356 -> [w360]
                  tunnel: w354 -> [w363] mode=indexing
                  tunnel: [w358] -> w353 mode=indexing
                  tunnel: [w359] -> w351 mode=indexing
                  tunnel: [w364] -> w352 mode=indexing
                  n164 = call-dynamic "check_is_moving.vi"("error in (no error)"=w360, "_stage in"=w363) -> ("error out"=w361:errorcluster, "_stage out"=w362:refnum<class "_stage.lvclass">)  [unwired: 7 in, 1 out]
                  n165 = call-dynamic "Read is moving_.vi"("error in (no error)"=w361, "_stage in"=w362) -> ("error out"=w365:errorcluster, "is moving?"=w364:bool, "_stage out"=w366:refnum<class "_stage.lvclass">)  [unwired: 7 in]
                  n166 = call-dynamic "get_curr_position.vi"("error in (no error)"=w365, "_stage in"=w366) -> ("error out"=w357:errorcluster, "readback position"=w367:dbl[], "_stage out"=w358:refnum<class "_stage.lvclass">)  [unwired: 7 in]
                  n167 = Index Array(array=w367) -> (element=w359:dbl)  [unwired: 1 in]
                }
              }
              frame True {
                # "set readback position as first stage position"
                n168 = for {
                  tunnel: w373 -> [w386] mode=indexing
                  tunnel: [w377] -> w371 mode=indexing
                  tunnel: [w375] -> w369 mode=indexing
                  shift-right: [w376] -> w370
                  shift-left: w372 -> [w385]
                  tunnel: [w374] -> w368 mode=indexing
                  n169 = call-dynamic "check_is_moving.vi"("error in (no error)"=w385, "_stage in"=w386) -> ("error out"=w383:errorcluster, "Numeric"=w374:dbl, "_stage out"=w384:refnum<class "_stage.lvclass">)  [unwired: 7 in]
                  n170 = Build Array(w374) -> (w382:dbl[])
                  n171 = call-dynamic "Write pos_curr.vi"("error in (no error)"=w383, "set_pos"=w382, "_stage in"=w384) -> ("error out"=w380:errorcluster, "_stage out"=w381:refnum<class "_stage.lvclass">)  [unwired: 7 in]
                  n172 = call-dynamic "check_is_moving.vi"("error in (no error)"=w380, "_stage in"=w381) -> ("error out"=w378:errorcluster, "_stage out"=w379:refnum<class "_stage.lvclass">)  [unwired: 7 in, 1 out]
                  n173 = call-dynamic "Read is moving_.vi"("error in (no error)"=w378, "_stage in"=w379) -> ("error out"=w376:errorcluster, "is moving?"=w375:bool, "_stage out"=w377:refnum<class "_stage.lvclass">)  [unwired: 7 in]
                }
                n174 = local write "stage position(s)"(w368) -> ()
              }
            }
            "stage position(s) readback" <- w336
            n175 = Not(x=w340) -> (.not. x?=w339:bool)
            n176 = Wait (ms)(milliseconds to wait=u32 150) -> ()  [unwired: 1 out]
            n177 = local write "is moving?"(w341) -> ()
            n178 = property class="_camera.lvclass"(reference=w350, error in=w347, "stage positions"=w336) -> (reference out=w349:refnum<class "_camera.lvclass">, error out=w348:errorcluster)
          }
          frame Error {
            n179 = Bundle(cluster=w394, "state"=state."stop" ("element")) -> (w392:cluster{"state":T4, "value":variant})  [unwired: 1 in]
            n180 = Enqueue Element(queue=w400, element=w392, error in (no error)=w399) -> ()  [unwired: 1 in, 3 out]
            n181 = Not(x=w388) -> (.not. x?=w387:bool)
            n182 = One Button Dialog(message="timeout caught an error", button name ("OK")="Exit and tell me what's up!") -> ()  [unwired: 1 out]
          }
        }
        "Boolean" <- w323
        n183 = local write "timed out?"(w321) -> ()
        "timed out?" <- w322
      }
      frame "hw_init" {
        n184 = flat-sequence {
          tunnel: w431 -> [w453]
          tunnel: w429 -> [w456]
          tunnel: w428 -> [w452]
          tunnel: [w450] -> w427
          tunnel: [w456] -> w426
          tunnel: [w455] -> w423
          tunnel: w422 -> [w455]
          tunnel: w421 -> [w454]
          tunnel: [w454] -> w420
          tunnel: [w451] -> w417
          tunnel: w402 -> [w449]
          tunnel: [w469] -> w425
          tunnel: [w470] -> w430
          tunnel: w427 -> [w470]
          tunnel: w426 -> [w469]
          tunnel: [w465] -> w424
          tunnel: w423 -> [w467]
          tunnel: w420 -> [w466]
          tunnel: [w464] -> w419
          tunnel: [w468] -> w418
          tunnel: w417 -> [w468]
          frame #0 {
            n185 = for {
              tunnel: w453 -> [w463] mode=indexing
              tunnel: [w458] -> w450 mode=indexing
              shift-right: [w457] -> w451
              shift-left: w452 -> [w462]
              i -> [w459]
              n186 = call-dynamic "set_params.vi"("_stage in"=w463, "error in (no error)"=w462) -> ("_stage out"=w461:refnum<class "_stage.lvclass">, "error out"=w460:errorcluster)  [unwired: 7 in]
              n187 = call-dynamic "Write stage num.vi"("error in (no error)"=w460, "stage num"=w459, "_stage in"=w461) -> ("error out"=w457:errorcluster, "_stage out"=w458:refnum<class "_stage.lvclass">)  [unwired: 7 in]
            }
            n188 = property class="_dataProcessing.lvclass"(reference=w449, "measurement type"="TA") -> ()  [unwired: 1 in, 2 out]
          }
          frame #1 {
            n189 = call-dynamic "set_params.vi"("error in (no error)"=w466, "_camera in"=w467) -> ("error out"=w464:errorcluster, "_camera out"=w465:refnum<class "_camera.lvclass">)  [unwired: 8 in]
          }
        }
        n190 = Bundle(cluster=w405, "state"=state."dat_send_to_process") -> (w407:cluster{"state":T4, "value":variant})  [unwired: 1 in]
        n191 = Enqueue Element(queue=w403, element=w407, error in (no error)=w404) -> ()  [unwired: 1 in, 3 out]
        n192 = call-dynamic "init_hw.vi"("error in (no error)"=w419, "_camera in"=w424) -> ("error out"=w434:errorcluster, "success ?"=w410:bool, "_camera out"=w436:refnum<class "_camera.lvclass">)  [unwired: 7 in]
        n193 = for {
          tunnel: w430 -> [w447] mode=indexing
          tunnel: [w446] -> w411 mode=indexing
          tunnel: [w445] -> w416 mode=indexing
          shift-right: [w444] -> w415
          shift-left: w418 -> [w443]
          n194 = call-dynamic "init_hw.vi"("error in (no error)"=w443, "_stage in"=w447) -> ("error out"=w444:errorcluster, "Boolean"=w446:bool, "_stage out"=w445:refnum<class "_stage.lvclass">)  [unwired: 7 in]
        }
        "Stage(s) initialized" <- w411
        n195 = Build Array(w410) -> (→"Camera initialised?":bool[])
        n196 = property class="_camera.lvclass"(reference=w436, error in=w434) -> (reference out=w435:refnum<class "_camera.lvclass">, error out=w433:errorcluster, "camera name and version"=→"camera name, version":string)
        n197 = for {
          tunnel: w416 -> [w442] mode=indexing
          tunnel: [w440] -> w414 mode=indexing
          shift-right: [w439] -> w413
          shift-left: w415 -> [w441]
          tunnel: [w438] -> w412 mode=indexing
          n198 = call-dynamic "Read stage name and version.vi"("error in (no error)"=w441, "_stage in"=w442) -> ("error out"=w439:errorcluster, "stage name and version"=w438:string, "_stage out"=w440:refnum<class "_stage.lvclass">)  [unwired: 7 in]
        }
        n199 = Bundle By Name(cluster=w425, "command"=data_process."init") -> (w408:T11)
        n200 = property on="stage name(s)" class="LstBox (strict)"("Item Names"=w412) -> ()  [unwired: 2 in, 2 out]
        "vi running?" <- TRUE
      }
      frame "sw_init" {
        w471 = bool[] [TRUE, TRUE, TRUE, FALSE]
        n201 = To Variant(anything=w471) -> (Variant=w472:variant)
        n202 = Bundle(cluster=w473, "state"=state."dat_update_save_type", "value"=w472) -> (w477:cluster{"state":T4, "value":variant})
        n203 = Enqueue Element(queue=w475, element=w477, error in (no error)=w474) -> ()  [unwired: 1 in, 3 out]
        n204 = property on="save type" class="Arr (strict)"("Value"=w471) -> ()  [unwired: 2 in, 2 out]
      }
      frame "cam_single_acq" {
        n205 = local read "is moving?"() -> (w491:bool[])
        n206 = Equal To 0?(x="move stage") -> (x = 0?=w484:bool)
        n207 = Or Array Elements(Boolean array=w491) -> (logical OR=w487:bool)
        n208 = And(x=w487, y=w484) -> (x .and. y?=w486:bool)
        n209 = case shown="False" w486 {
          tunnel: w500 -> [w522 w534]
          tunnel: w499 -> [w521 w533]
          tunnel: w498 -> [w520 w529]
          tunnel: [w516 w534] -> w497
          tunnel: [w514 w533] -> w496
          tunnel: w495 -> [w513 w532]
          tunnel: w494 -> [w512 w531]
          tunnel: [w511 w531] -> w493
          tunnel: [w509 w532] -> w492
          tunnel: w490 -> [w503 w542]
          tunnel: w489 -> [w502 w541]
          tunnel: w488 -> [w504 w535]
          tunnel: [w507 w529] -> w483
          frame False {
            n210 = call-dynamic "get_single_acq.vi"("error in (no error)"=w521, "_camera in"=w522) -> ("error out"=w515:errorcluster, "trigger"=w508:bool[][], "raw data"=w519:i32[][][], "_camera out"=w518:refnum<class "_camera.lvclass">)  [unwired: 6 in]
            n211 = property class="_camera.lvclass"(reference=w518, error in=w515) -> (reference out=w516:refnum<class "_camera.lvclass">, error out=w514:errorcluster, "wavelength"=w517:dbl[])
            n212 = for {
              tunnel: w513 -> [w528] mode=indexing
              tunnel: [w523] -> w510 mode=indexing
              tunnel: [w525] -> w509 mode=indexing
              shift-right: [w526] -> w511
              shift-left: w512 -> [w527]
              n213 = call-dynamic "get_curr_position.vi"("error in (no error)"=w527, "_stage in"=w528) -> ("error out"=w526:errorcluster, "readback position"=w524:dbl[], "_stage out"=w525:refnum<class "_stage.lvclass">)  [unwired: 7 in]
              n214 = Index Array(array=w524) -> (element=w523:dbl)  [unwired: 1 in]
            }
            n215 = Bundle(cluster=w504, "state"=state."dat_send_to_process") -> (w506:cluster{"state":T4, "value":variant})  [unwired: 1 in]
            n216 = Enqueue Element At Opposite End(queue=w502, element=w506, error in (no error)=w503) -> ()  [unwired: 1 in, 3 out]
            n217 = local write "stage position(s) readback"(w510) -> ()
            n218 = Bundle By Name(cluster=w520, "command"=data_process."process", "wavelength"=w517, "raw data"=w519, "trigger"=w508) -> (w507:T11)
          }
          frame True {
            # "need to reverse order when enqueuing at opposite end !!!!!!"
            n219 = Bundle(cluster=w535, "state"=state."cam_single_acq") -> (w540:cluster{"state":T4, "value":variant})  [unwired: 1 in]
            n220 = Enqueue Element At Opposite End(queue=w541, element=w540, error in (no error)=w542) -> (queue out=w537:refnum<queue>, error out=w536:errorcluster)  [unwired: 1 in, 1 out]
            n221 = Bundle(cluster=w535, "state"=state."timeout") -> (w538:cluster{"state":T4, "value":variant})  [unwired: 1 in]
            n222 = Enqueue Element At Opposite End(queue=w537, element=w538, error in (no error)=w536) -> ()  [unwired: 1 in, 3 out]
          }
        }
      }
      frame "cam_get_bg" {
        n223 = call-dynamic "get_single_acq.vi"("error in (no error)"=w548, "_camera in"=w553) -> ("error out"=w547:errorcluster, "raw data"=w550:i32[][][], "_camera out"=w552:refnum<class "_camera.lvclass">)  [unwired: 6 in, 1 out]
        n224 = for {
          tunnel: [w556] -> w549 mode=indexing
          tunnel: w550 -> [w554] mode=indexing
          n225 = Transpose 2D Array(2D array=w554) -> (transposed array=w555:i32[][])
          n226 = for {
            tunnel: w555 -> [w558] mode=indexing
            tunnel: [w557] -> w556 mode=indexing
            n227 = call-poly <vilib>:"Mean.vi"("X"=w558) -> ("mean"=w557:dbl)  [unwired: 1 out]
          }
        }
        n228 = property class="_camera.lvclass"(reference=w552, error in=w547, "background"=w549) -> (reference out=w551:refnum<class "_camera.lvclass">, error out=w546:errorcluster)
      }
      frame "cam_rst_bg" {
        n229 = property class="_camera.lvclass"(reference=w566, error in=w563, "background"=i32[][] []) -> (reference out=w565:refnum<class "_camera.lvclass">, error out=w562:errorcluster)
      }
      frame "cam_cnt_acq" {
        # "need to make sure that safe flag is false"
        n230 = Bundle(cluster=w571, "state"=state."cam_single_acq") -> (w577:cluster{"state":T4, "value":variant})  [unwired: 1 in]
        n231 = Enqueue Element(queue=w585, element=w577, error in (no error)=w584) -> (queue out=w583:refnum<queue>, error out=w582:errorcluster)  [unwired: 1 in, 1 out]
        n232 = Bundle(cluster=w571, "state"=state."timeout" ("element")) -> (w575:cluster{"state":T4, "value":variant})  [unwired: 1 in]
        n233 = Enqueue Element(queue=w583, element=w575, error in (no error)=w582) -> (queue out=w572:refnum<queue>, error out=w573:errorcluster)  [unwired: 1 in, 1 out]
        n234 = property on="history length" class="DigNum (strict)"("Value"=30 ("history length")) -> ()  [unwired: 2 in, 2 out]
        n235 = Bundle(cluster=w571, "state"=state."cam_cnt_acq") -> (w574:cluster{"state":T4, "value":variant})  [unwired: 1 in]
        n236 = Enqueue Element(queue=w572, element=w574, error in (no error)=w573) -> ()  [unwired: 1 in, 3 out]
      }
      frame "cam_set_wl" {
        n237 = Variant To Data(type=TRUE, Variant=w598) -> (data=w597:bool)  [unwired: 1 in, 1 out]
        n238 = property class="_camera.lvclass"(reference=w607, error in=w606) -> (reference out=w605:refnum<class "_camera.lvclass">, "wavelength"=w604:dbl[])  [unwired: 1 out]
        n239 = Array Size(array=w604) -> (size(s)=w603:i32)
        n240 = case shown="True" w597 {
          tunnel: w603 -> [w617 w625]
          tunnel: [w616 w620] -> w591
          tunnel: [w616 w624] -> w587
          tunnel: [w616 w623] -> w590
          tunnel: [w616 w619] -> w599
          frame False {
            n241 = for {
              N: w617 -> [_]
              tunnel: [w618] -> w616 mode=indexing
              i -> [w618]
            }
          }
          frame True {
            n242 = Sort 1D Array(array="wavelength \n(calibration value)") -> (sorted array=w622:dbl[])
            n243 = case shown="False" "mirror?" {
              tunnel: w622 -> [w663 w665]
              tunnel: [w663 w664] -> w619
              frame False {
              }
              frame True {
                n244 = Reverse 1D Array(array=w665) -> (reversed array=w664:dbl[])
              }
            }
            n245 = Sort 1D Array(array="pixel/index") -> (sorted array=w620:u16[])
            n246 = disable-structure shown="Enabled" {
              disable-tunnel: "parameter bounds" -> [w640 _]
              disable-tunnel: "method" -> [w639 _]
              disable-tunnel: w625 -> [w634 w653]
              disable-tunnel: [w633 w649] -> w624
              disable-tunnel: [w632 w650] -> w623
              disable-tunnel: w619 -> [w631 w659]
              disable-tunnel: w620 -> [w630 w660]
              frame Disabled {
                n247 = call <vilib>:"Power Fit.vi"("Y"=w631, "X"=w630, "method"=w639, "parameter bounds"=w640) -> ("Best Power Fit"=w638:dbl[], "amplitude"=w637:dbl, "power"=w636:dbl, "offset"=w635:dbl)  [unwired: 6 in, 2 out]
                "amplitude" <- w637
                "power" <- w636
                "offset" <- w635
                n248 = for {
                  N: w634 -> [_]
                  tunnel: w638 -> [_]
                  tunnel: w637 -> [w647]
                  tunnel: w636 -> [w648]
                  tunnel: w635 -> [w644]
                  tunnel: [w643] -> w632 mode=indexing
                  tunnel: [w642] -> w633 mode=indexing
                  i -> [w642]
                  n249 = Increment(x=w642) -> (x+1=w641:i32)
                  n250 = Power Of X(1:w641, 2:w648) -> (0:w646:dbl)
                  n251 = Multiply(x=w647, y=w646) -> (x*y=w645:dbl)
                  n252 = Add(x=w645, y=w644) -> (x+y=w643:dbl)
                }
              }
              frame Enabled {
                n253 = call-poly <vilib>:"Nonlinear Curve Fit.vi"("Y"=w659, "initial parameters"="initial parameters", "X"=w660, "model description"=T19 {"model"="a1+a2/(x-a3)", "Parameters"=["a1", "a2", "a3"], "x"="x"}) -> ("best fit parameters"=w657:dbl[])  [unwired: 7 in, 4 out]
                "best fit parameters" <- w657
                n254 = for {
                  N: w653 -> [_]
                  tunnel: [w662] -> w649 mode=indexing
                  i -> [w662]
                }
                n255 = Index Array(array=w657) -> (element #1=w656:dbl, element #2=w655:dbl, element #3=w652:dbl)  [unwired: 3 in]
                n256 = Subtract(x=w649, y=w652) -> (x-y=w654:dbl[])
                n257 = Divide(x=w655, y=w654) -> (x/y=w651:dbl[])
                n258 = Add(x=w656, y=w651) -> (x+y=w650:dbl[])
              }
            }
          }
        }
        n259 = local read "pixel/index"() -> (w586:u16[])
        n260 = for {
          tunnel: w586 -> [w615] mode=indexing
          tunnel: w590 -> [w614]
          tunnel: [w613] -> w594 mode=indexing
          n261 = Index Array(array=w614, index=w615) -> (element=w613:dbl)
        }
        "wavelength (fitted)" <- w594
        n262 = local read "wavelength \n(calibration value)"() -> (w595:dbl[])
        n263 = Subtract(x=w590, y=w590) -> (x-y=w589:dbl[])
        n264 = property class="_camera.lvclass"(reference=w605, "wavelength"=w590) -> (reference out=w612:refnum<class "_camera.lvclass">, error out=w611:errorcluster)  [unwired: 1 in]
        n265 = Bundle(w591, w599) -> (w602:cluster{i32[], dbl[]})  [unwired: 1 in]
        n266 = Bundle(w587, w590) -> (w601:cluster{i32[], dbl[]})  [unwired: 1 in]
        n267 = Bundle(w587, w589) -> (w588:cluster{i32[], dbl[]})  [unwired: 1 in]
        n268 = Subtract(x=w595, y=w594) -> (x-y=w593:dbl[])
        n269 = Bundle("pixel/index"=w586, w593) -> (w592:cluster{"pixel/index":u16[], dbl[]})  [unwired: 1 in]
        n270 = Build Array(w602, w601, w592, w588) -> (→"wavelength fit":cluster{"pixel/index":i32[], dbl[]}[])
      }
      frame "stg_set_pos" {
        n271 = Variant To Data(type=0, Variant=w670) -> (data=w667:i32)  [unwired: 1 in, 1 out]
        "value" <- w667
        n272 = flat-sequence {
          tunnel: w667 -> [w683]
          tunnel: [w683] -> w668
          frame #0 {
            n273 = local read "is moving?"() -> (w686:bool[])
            n274 = Replace Array Subset(array=w686, new element=TRUE ("new element/subarray"), index=w683) -> (→"is moving?":bool[])
          }
        }
        n275 = Index Array(array=w677, index=w668) -> (element=w678:refnum<class "_stage.lvclass">)
        n276 = Index Array(array="stage position(s)", index=w668) -> (element=w676:dbl)
        n277 = Build Array(w676) -> (w675:dbl[])
        n278 = property class="_camera.lvclass"(reference=w681, "stage positions"="stage position(s)") -> (reference out=w680:refnum<class "_camera.lvclass">)  [unwired: 1 in, 1 out]
        n279 = call-dynamic "set_new_position.vi"("error in (no error)"=w679, "set_pos"=w675, "_stage in"=w678) -> ("error out"=w671:errorcluster, "_stage out"=w672:refnum<class "_stage.lvclass">)  [unwired: 7 in]
        n280 = Replace Array Subset(array=w677, new element=w672, index=w668) -> (w674:refnum<class "_stage.lvclass">[])
      }
      frame "stg_home" {
      }
      frame "scn_load_step_file" {
        n281 = Variant To Data(type=path "", Variant=w698) -> (data=w696:path)  [unwired: 1 in, 1 out]
        n282 = call-poly <vilib>:"Read Delimited Spreadsheet.vi"("file path (dialog if empty)"=w696, "transpose? (F)"=TRUE) -> ("first row"=w692:dbl[])  [unwired: 8 in, 5 out]
        n283 = Bundle By Name(cluster=w694, "scn_step_time_dly"=w692) -> (w693:T11)
      }
      frame "scn_init" {
        w705 = 0 ("scn_iter")
        n284 = Unbundle By Name(w724) -> ("scn_step_time_dly"=w704:dbl[])
        n285 = Get Date/Time In Seconds() -> (seconds since 1Jan1904=w712:timestamp)
        n286 = Empty Array?(array=w704) -> (empty?=w728:bool)
        n287 = Format Date/Time String(time format string (%c)="%Y%m%d", seconds (now)=w712) -> (date/time string=w714:string)  [unwired: 1 in]
        n288 = Array Size(array=w704) -> (size(s)=w703:i32)
        n289 = Build Path(base path="data folder", name or relative path=w714) -> (appended path=w715:path)
        n290 = case shown="False" w728 {
          tunnel: w727 -> [w738 w747]
          tunnel: w726 -> [w737 w746]
          tunnel: w725 -> [w736 w741]
          tunnel: w703 -> [w735 _]
          frame False {
            n291 = Add(x=w735, y=10) -> (x+y=w734:i32)
            n292 = Bundle(cluster=w736, "state"=state."scn_next_step") -> (w740:cluster{"state":T4, "value":variant})  [unwired: 1 in]
            n293 = Enqueue Element(queue=w738, element=w740, error in (no error)=w737) -> ()  [unwired: 1 in, 3 out]
            n294 = property on="history length" class="DigNum (strict)"("Value"=w734) -> ()  [unwired: 2 in, 2 out]
          }
          frame True {
            n295 = Bundle(cluster=w741, "state"=state."scn_load_step_file") -> (w749:cluster{"state":T4, "value":variant})  [unwired: 1 in]
            n296 = Enqueue Element(queue=w747, element=w749, error in (no error)=w746) -> (queue out=w743:refnum<queue>, error out=w742:errorcluster)  [unwired: 1 in, 1 out]
            n297 = Bundle(cluster=w741, "state"=state."scn_init") -> (w745:cluster{"state":T4, "value":variant})  [unwired: 1 in]
            n298 = Enqueue Element(queue=w743, element=w745, error in (no error)=w742) -> ()  [unwired: 1 in, 3 out]
          }
        }
        n299 = Build Path(base path=w715, name or relative path="Experiment") -> (appended path=w717:path)
        n300 = Build Path(base path=w717, name or relative path="sample") -> (appended path=w707:path)
        n301 = local read "N scans"() -> (w721:u16)
        n302 = Path To String(path=w707) -> (string=w711:string)
        n303 = Format Into String(format string="_scan%03d" ("initial string"), w705) -> (resulting string=w708:string)  [unwired: 2 in, 1 out]
        n304 = property on="progress" class="Slide (strict)"("Scale.Maximum"=w721, "Scale.Minimum"=0.0 ("Scale.Range:Minimum")) -> ()  [unwired: 2 in, 2 out]
        n305 = Concatenate Strings(w711, w708) -> (w710:string)
        n306 = String To Path(string=w710) -> (path=w706:path)
        n307 = Bundle By Name(cluster=w724, "scn_step"=-1, "scn_iter"=w705, "save path"=w706) -> (w722:T11)
        n308 = local write "current scan"(w705) -> ()
      }
      frame "scn_next_step" {
        n309 = Unbundle By Name(w758) -> ("scn_step_time_dly"=w755:dbl[], "scn_step"=w754:i32, "scn_iter"=→"current scan" →"progress":i32)
        "scan progress" <- w754
        n310 = local read "t0 position(s)"() -> (w750:dbl[])
        n311 = Array Size(array=w755) -> (size(s)=w753:i32)
        n312 = Greater?(x=w753, y=w754) -> (0:w756:bool)
        n313 = case shown="True" w756 {
          tunnel: w761 -> [w770 w799]
          tunnel: w760 -> [w769 w798]
          tunnel: w759 -> [w768 w784]
          tunnel: w758 -> [w766 w782]
          tunnel: [w766 w781] -> w757
          tunnel: w755 -> [_ w779]
          tunnel: w754 -> [_ w778]
          tunnel: w750 -> [_ w776]
          frame False {
            n314 = Bundle(cluster=w768, "state"=state."scn_next_iter") -> (w771:cluster{"state":T4, "value":variant})  [unwired: 1 in]
            n315 = Enqueue Element(queue=w770, element=w771, error in (no error)=w769) -> ()  [unwired: 1 in, 3 out]
          }
          frame True {
            # "find better solution"
            n316 = Index Array(array=w776) -> (element=w773:dbl)  [unwired: 1 in]
            n317 = Index Array(array=w779, index=w778) -> (element=w775:dbl)
            n318 = Increment(x=w778) -> (x+1=w780:i32)
            n319 = Bundle(cluster=w784, "state"=state."stg_set_pos") -> (w797:cluster{"state":T4, "value":variant})  [unwired: 1 in]
            n320 = Enqueue Element(queue=w799, element=w797, error in (no error)=w798) -> (queue out=w794:refnum<queue>, error out=w793:errorcluster)  [unwired: 1 in, 1 out]
            n321 = case shown="False" "is stage reversed?" {
              tunnel: w775 -> [w802 w805]
              tunnel: [w800 w804] -> w774
              tunnel: w773 -> [w801 w803]
              frame False {
                n322 = Add(x=w801, y=w802) -> (x+y=w800:dbl)
              }
              frame True {
                n323 = Subtract(x=w803, y=w805) -> (x-y=w804:dbl)
              }
            }
            n324 = Bundle(cluster=w784, "state"=state."cam_single_acq") -> (w795:cluster{"state":T4, "value":variant})  [unwired: 1 in]
            n325 = Build Array(w774) -> (w777:dbl[])
            n326 = Bundle By Name(cluster=w782, "scn_step"=w780) -> (w781:T11)
            n327 = Enqueue Element(queue=w794, element=w795, error in (no error)=w793) -> (queue out=w790:refnum<queue>, error out=w789:errorcluster)  [unwired: 1 in, 1 out]
            n328 = property on="stage position(s)" class="Arr (strict)"("Value"=w777) -> ()  [unwired: 2 in, 2 out]
            n329 = Bundle(cluster=w784, "state"=state."timeout") -> (w791:cluster{"state":T4, "value":variant})  [unwired: 1 in]
            n330 = Enqueue Element(queue=w790, element=w791, error in (no error)=w789) -> (queue out=w786:refnum<queue>, error out=w785:errorcluster)  [unwired: 1 in, 1 out]
            n331 = Bundle(cluster=w784, "state"=state."scn_next_step") -> (w787:cluster{"state":T4, "value":variant})  [unwired: 1 in]
            n332 = Enqueue Element(queue=w786, element=w787, error in (no error)=w785) -> ()  [unwired: 1 in, 3 out]
          }
        }
        n333 = property on="scan progress" class="Slide (strict)"("Scale.Maximum"=w753, "Scale.Minimum"=0.0 ("Scale.Range:Minimum")) -> ()  [unwired: 2 in, 2 out]
      }
      frame "scn_next_iter" {
        n334 = Unbundle By Name(w808) -> ("save path"=w807:path, "scn_iter"=w806:i32)
        n335 = Unbundle By Name(w808) -> ("scn_iter"=w817:i32)
        n336 = Less?(x=w817, y="N scans") -> (x < y?=w818:bool)
        n337 = case shown="False" w818 {
          tunnel: w808 -> [w821 w844]
          tunnel: w817 -> [_ _]
          tunnel: [w821 w842] -> w816
          tunnel: w815 -> [w823 w839]
          tunnel: w814 -> [w822 w838]
          tunnel: w813 -> [_ w837]
          tunnel: w807 -> [_ w836]
          tunnel: w806 -> [_ w824]
          frame False {
            n338 = Flush Queue(queue=w823, error in (no error)=w822) -> ()  [unwired: 3 out]
            n339 = property on="scan" class="Bool (strict)"("Value"=FALSE ("scan")) -> ()  [unwired: 2 in, 2 out]
          }
          frame True {
            n340 = Increment(x=w824) -> (x+1=w831:i32)
            n341 = Strip Path(path=w836) -> (stripped path=w826:path, name=w830:string)
            n342 = String Length(string=w830) -> (length=w835:i32)
            n343 = Bundle(cluster=w837, "state"=state."scn_next_step") -> (w841:cluster{"state":T4, "value":variant})  [unwired: 1 in]
            n344 = Subtract(x=w835, y=3) -> (x-y=w833:i32)
            n345 = String Subset(string=w830, length (rest)=w833) -> (substring=w832:string)  [unwired: 1 in]
            n346 = Enqueue Element(queue=w839, element=w841, error in (no error)=w838) -> ()  [unwired: 1 in, 3 out]
            n347 = Format Into String(format string="%03d", w831) -> (resulting string=w828:string)  [unwired: 2 in, 1 out]
            n348 = Concatenate Strings(w832, w828) -> (w827:string)
            n349 = Build Path(base path=w826, name or relative path=w827) -> (appended path=w825:path)
            n350 = Bundle By Name(cluster=w844, "scn_step"=-1, "scn_iter"=w831, "save path"=w825) -> (w842:T11)
          }
        }
      }
      frame "dat_update_save_flag" {
        n351 = Variant To Data(type=FALSE, Variant=w847) -> (data=w845:bool)  [unwired: 1 in, 1 out]
        n352 = Bundle By Name(cluster=w853, "save flag"=w845) -> (w852:T11)
      }
      frame "dat_update_save_type" {
        n353 = Variant To Data(type=bool[] [], Variant=w857) -> (data=w858:bool[])  [unwired: 1 in, 1 out]
        n354 = Bundle By Name(cluster=w860, "save type"=w858) -> (w859:T11)
      }
      frame "dat_save_raw" {
        n355 = To Variant(anything=bool[] [FALSE, FALSE, FALSE, TRUE]) -> (Variant=w890:variant)
        n356 = Bundle(cluster=w882, "state"=state."dat_update_save_type", "value"=w890) -> (w893:cluster{"state":T4, "value":variant})
        n357 = local read "data folder"() -> (w866:path)
        n358 = Enqueue Element(queue=w892, element=w893, error in (no error)=w891) -> (queue out=w886:refnum<queue>, error out=w885:errorcluster)  [unwired: 1 in, 1 out]
        n359 = Get Date/Time In Seconds() -> (seconds since 1Jan1904=w869:timestamp)
        n360 = Format Date/Time String(time format string (%c)="%Y%m%d", seconds (now)=w869) -> (date/time string=w871:string)  [unwired: 1 in]
        n361 = Build Path(base path=w866, name or relative path=w871) -> (appended path=w868:path)
        n362 = Bundle(cluster=w882, "state"=state."cam_single_acq") -> (w887:cluster{"state":T4, "value":variant})  [unwired: 1 in]
        n363 = Enqueue Element(queue=w886, element=w887, error in (no error)=w885) -> (queue out=w881:refnum<queue>, error out=w880:errorcluster)  [unwired: 1 in, 1 out]
        n364 = Build Path(base path=w868, name or relative path="raw_acquisition") -> (appended path=w865:path)
        n365 = Build Path(base path=w865, name or relative path="raw") -> (appended path=w864:path)
        n366 = Unbundle By Name(w873) -> ("save type"=w877:bool[])
        n367 = Bundle By Name(cluster=w873, "save path"=w864) -> (w872:T11)
        n368 = To Variant(anything=w877) -> (Variant=w876:variant)
        n369 = Bundle(cluster=w882, "state"=state."dat_update_save_type", "value"=w876) -> (w883:cluster{"state":T4, "value":variant})
        n370 = Enqueue Element(queue=w881, element=w883, error in (no error)=w880) -> ()  [unwired: 1 in, 3 out]
      }
      frame "dat_send_to_process" {
        n371 = Variant To Data(type=TRUE, Variant=w901) -> (data=w899:bool, error out=w898:errorcluster)  [unwired: 1 in]
        n372 = case shown="No Error" w898 {
          tunnel: w899 -> [w906 _]
          frame No Error {
            n373 = case shown="True" w906 {
              selector: w906 -> [_ w907]
              frame False {
              }
              frame True {
                "Boolean 2" <- w907
              }
            }
          }
          frame Error {
          }
        }
        n374 = Enqueue Element(queue=w897, element=w895, error in (no error)=w896) -> ()  [unwired: 1 in, 3 out]
      }
      frame "dat_save_wl_to_ini" {
        w911 = ""
        w908 = TRUE ("replace all? (F)")
        w956 = "values" ("section")
        w970 = "calibration" ("section")
        # "overwrite config values and then eliminated stupid \"quotes\""
        n375 = local read "best fit parameters"() -> (w974:dbl[])
        n376 = call <vilib>:"Application Directory.vi"() -> ("Application Directory"=w978:path)
        n377 = local read "wavelength \n(calibration value)"() -> (w950:dbl[])
        n378 = Build Path(base path=w978, name or relative path="cameras\\spectral_calibration.ini") -> (appended path=w938:path)
        n379 = call <vilib>:"Open Config Data.vi"("create file if necessary (T)"=FALSE, "configuration file path"=w938) -> ("error out"=w972:errorcluster, "refnum"=w973:T10)  [unwired: 7 in, 1 out]
        n380 = Index Array(array=w974) -> (element #1=w971:dbl, element #2=w963:dbl, element #3=w962:dbl)  [unwired: 3 in]
        n381 = call-poly <vilib>:"Write Key.vi"("section"=w970, "error in (no error)"=w972, "value"=w971, "key"="amp", "refnum"=w973) -> ("error out"=w966:errorcluster, "refnum out"=w969:T10)  [unwired: 4 in, 1 out]
        n382 = Array To Spreadsheet String(delimiter (Tab)=",", array=w950, 3:"%.0f" ("format string")) -> (spreadsheet string=w924:string)
        n383 = call-poly <vilib>:"Write Key.vi"("section"=w970, "error in (no error)"=w966, "value"=w963, "key"="pow", "refnum"=w969) -> ("error out"=w967:errorcluster, "refnum out"=w968:T10)  [unwired: 4 in, 1 out]
        n384 = local read "pixel/index"() -> (w954:u16[])
        n385 = call-poly <vilib>:"Write Key.vi"("section"=w970, "error in (no error)"=w967, "value"=w962, "key"="off", "refnum"=w968) -> ("error out"=w960:errorcluster, "refnum out"=w961:T10)  [unwired: 4 in, 1 out]
        n386 = Search and Replace String(replace all?=TRUE ("replace all? (F)"), input string=w924, search string="\n", replace string="" ("replace string (\"\")")) -> (result string=w922:string)  [unwired: 4 in, 3 out]
        n387 = Array To Spreadsheet String(delimiter (Tab)=",", array=w954, 3:"%.0f" ("format string")) -> (spreadsheet string=w951:string)
        n388 = call-poly <vilib>:"Write Key.vi"("write raw string? (F)"=TRUE, "section"=w956, "error in (no error)"=w960, "value"=w951, "key"="pix", "refnum"=w961) -> ("error out"=w957:errorcluster, "refnum out"=w958:T10)  [unwired: 3 in, 1 out]
        n389 = call-poly <vilib>:"Write Key.vi"("write raw string? (F)"=TRUE, "section"=w956, "error in (no error)"=w957, "value"=w922, "key"="wls", "refnum"=w958) -> ("error out"=w947:errorcluster, "refnum out"=w944:T10)  [unwired: 3 in, 1 out]
        n390 = call <vilib>:"Close Config Data.vi"("error in (no error)"=w947, "refnum"=w944) -> ("error out"=w936:errorcluster)  [unwired: 8 in, 1 out]
        n391 = Open/Create/Replace File(file path (use dialog)=w938, error in=w936, operation (0:open)=T20."open", access (0:read/write)=enum16{"read/write", "read-only", "write-only"}."read/write") -> (refnum out=w937:refnum<file>, error out=w933:errorcluster)  [unwired: 2 in, 1 out]
        n392 = Concatenate Strings("\n", "\"" ("string")) -> (w925:string)
        n393 = Read from Text File(file (use dialog)=w937, error in=w933) -> (refnum out=w929:refnum<file>, text=w943:string, error out=w941:errorcluster)  [unwired: 2 in, 1 out]
        n394 = Search and Replace String(replace all?=w908, input string=w943, search string=w925, replace string=w911, error in=w941) -> (result string=w917:string, error out=w916:errorcluster)  [unwired: 3 in, 2 out]
        n395 = Search and Replace String(replace all?=w908, input string=w917, search string="\"", replace string=w911, error in=w916) -> (result string=w914:string, error out=w913:errorcluster)  [unwired: 3 in, 2 out]
        n396 = call <vilib>:"Space Constant.vi"() -> ("String"=w912:string)
        n397 = Search and Replace String(replace all?=w908, input string=w914, search string=w912, replace string=w911, error in=w913) -> (result string=w910:string, error out=w909:errorcluster)  [unwired: 3 in, 2 out]
        n398 = Set File Size(4:w909, 6:i64 0 ("size (in bytes)"), 7:w929) -> (0:w928:errorcluster, 3:w927:refnum<file>)
        n399 = Set File Position(offset (in bytes) (0)=i64 0, refnum=w927, error in=w928) -> (refnum out=w931:refnum<file>, error out=w930:errorcluster)  [unwired: 1 in]
        n400 = Write to Text File(file (use dialog)=w931, text=w910, error in=w930) -> (refnum out=w942:refnum<file>, error out=w940:errorcluster)  [unwired: 1 in, 1 out]
        n401 = Close File(refnum=w942, error in=w940) -> (error out=w939:errorcluster)  [unwired: 1 out]
        n402 = call <vilib>:"Simple Error Handler.vi"("error in (no error)"=w939) -> ()  [unwired: 4 in, 5 out]
      }
      frame "stop" {
        w1008 = TRUE
        n403 = for {
          tunnel: w1001 -> [w1013] mode=indexing
          tunnel: [w1010] -> w998 mode=indexing
          shift-right: [w1011] -> w999
          shift-left: w1000 -> [w1012]
          n404 = call-dynamic "close_hw.vi"("error in (no error)"=w1012, "_stage in"=w1013) -> ("error out"=w1011:errorcluster, "_stage out"=w1010:refnum<class "_stage.lvclass">)  [unwired: 8 in]
        }
        n405 = Bundle(cluster=w989, "state"=state."dat_send_to_process", "value"=TRUE) -> (w991:cluster{"state":T4, "value":variant})
        n406 = Enqueue Element(queue=w995, element=w991, error in (no error)=w994) -> (queue out=w992:refnum<queue>, error out=w993:errorcluster)  [unwired: 1 in, 1 out]
        n407 = call-dynamic "release_hw.vi"("error in (no error)"=w1004, "_camera in"=w1007) -> ("error out"=w1002:errorcluster, "_camera out"=w1006:refnum<class "_camera.lvclass">)  [unwired: 8 in]
        n408 = Release Queue(queue=w992, error in (no error)=w993) -> ()  [unwired: 1 in, 3 out]
        n409 = Bundle By Name(cluster=w1003, "command"=data_process."exit") -> (w985:T11)
        n410 = Build Array(FALSE ("camera initialized?")) -> (w996:bool[])
        n411 = Enqueue Element(queue=w987, element=w985, error in (no error)=w986) -> ()  [unwired: 1 in, 3 out]
        n412 = local write "Stage(s) initialized"(bool[] [FALSE] ("Stage(s) initialized")) -> ()
        n413 = local write "Camera initialised?"(w996) -> ()
        n414 = Not(x=w1008) -> (.not. x?=w1009:bool)
        n415 = local write "vi running?"(w1009) -> ()
      }
    }
    n416 = Merge Errors(w310, w308) -> (w309:errorcluster)
  }
  n417 = while {
    tunnel: w2 -> [w1018]
    tunnel: w1 -> [w1017]
    tunnel: w3 -> [w1014]
    stop <- w1016 stop-if-true
    # "Control"
    n418 = event shown="[9] \"save wl calibration to .ini\": Value Change" {
      selector: _ -> [_ _ _ _ _ _ _ _ _ _ _ _ _ _ _ _ _ _ _ _ _ _ _ _]
      dyn-events: _ -> [_ _ _ _ _ _ _ _ _ _ _ _ _ _ _ _ _ _ _ _ _ _ _ _]
      timeout: 10 -> [_ _ _ _ _ _ _ _ _ _ _ _ _ _ _ _ _ _ _ _ _ _ _ _]
      tunnel: w1018 -> [_ w1026 w1047 w1051 w1065 _ _ _ _ w1090 w1104 _ _ w1129 w1144 w1150 w1165 _ w1174 w1179 _ _ _ w1216]
      tunnel: w1017 -> [_ w1025 w1046 w1050 w1064 _ _ _ _ w1091 w1103 _ _ w1128 w1143 w1149 w1164 _ w1173 w1178 _ _ _ w1215]
      tunnel: [_ _ _ _ _ _ _ _ _ _ _ _ _ _ _ _ _ _ _ _ _ _ _ w1217] -> w1016
      tunnel: w1014 -> [_ w1027 w1045 w1048 w1062 _ _ _ _ w1089 w1099 _ _ w1130 w1142 w1148 w1166 _ w1171 w1180 _ _ _ w1214]
      event Timeout {
        n419 = event-data() -> ()  [unwired: 1 in, 3 out]
        n420 = Divide(x="diff", y=1.0) -> (x/y=w1020:dbl)
        n421 = Negate(x=w1020) -> (-x=w1019:dbl)
        n422 = property on="main graph" class="XYGraph (strict)"("ActYScl"=1 ("Active Y Scale"), "YScale.Maximum"=w1020, "YScale.Minimum"=w1019) -> ()  [unwired: 2 in, 2 out]
        n423 = property on="Intensity Chart" class="IntChart (strict)"("ZScale.Maximum"=w1020, "ZScale.Minimum"=w1019) -> ()  [unwired: 2 in, 2 out]
        n424 = property on="Intensity Graph" class="IntGraph (strict)"("ZScale.Maximum"=w1020, "ZScale.Minimum"=w1019) -> ()  [unwired: 2 in, 2 out]
      }
      event "calibrate wavelength": Value Change {
        n425 = event-data() -> ("NewVal"=w1024:bool)  [unwired: 1 in]
        n426 = case shown="False" w1024 {
          tunnel: w1027 -> [w1030 w1039]
          tunnel: w1026 -> [w1029 w1038]
          tunnel: w1025 -> [w1028 w1037]
          frame False {
            n427 = To Variant(anything=FALSE) -> (Variant=w1031:variant)
            n428 = Bundle(cluster=w1030, "state"=state."cam_set_wl" ("element"), "value"=w1031) -> (w1033:cluster{"state":T4, "value":variant})
            n429 = Enqueue Element(queue=w1029, element=w1033, error in (no error)=w1028) -> ()  [unwired: 1 in, 3 out]
          }
          frame True {
            n430 = To Variant(anything=TRUE) -> (Variant=w1035:variant)
            n431 = Bundle(cluster=w1039, "state"=state."cam_set_wl" ("element"), "value"=w1035) -> (w1040:cluster{"state":T4, "value":variant})
            n432 = Enqueue Element(queue=w1038, element=w1040, error in (no error)=w1037) -> ()  [unwired: 1 in, 3 out]
          }
        }
      }
      event "get_single_acq": Value Change {
        n433 = event-data() -> ("OldVal"=w1043:bool)  [unwired: 1 in]
        n434 = Bundle(cluster=w1045, "state"=state."cam_single_acq") -> (w1044:cluster{"state":T4, "value":variant})  [unwired: 1 in]
        n435 = Enqueue Element(queue=w1047, element=w1044, error in (no error)=w1046) -> ()  [unwired: 1 in, 3 out]
        n436 = property on="get_single_acq" class="Bool (strict)"("Value"=w1043) -> ()  [unwired: 2 in, 2 out]
      }
      event "get bg": Value Change {
        n437 = event-data() -> ("NewVal"=w1049:bool)  [unwired: 1 in]
        n438 = case shown="True" w1049 {
          tunnel: w1051 -> [w1056 w1061]
          tunnel: w1050 -> [w1055 w1060]
          tunnel: w1048 -> [w1054 w1059]
          frame False {
            n439 = Bundle(cluster=w1054, "state"=state."cam_rst_bg") -> (w1053:cluster{"state":T4, "value":variant})  [unwired: 1 in]
            n440 = Enqueue Element(queue=w1056, element=w1053, error in (no error)=w1055) -> ()  [unwired: 1 in, 3 out]
          }
          frame True {
            n441 = Bundle(cluster=w1059, "state"=state."cam_get_bg" ("element")) -> (w1057:cluster{"state":T4, "value":variant})  [unwired: 1 in]
            n442 = Enqueue Element(queue=w1061, element=w1057, error in (no error)=w1060) -> ()  [unwired: 1 in, 3 out]
          }
        }
      }
      event "cont acq": Value Change {
        n443 = event-data() -> ("NewVal"=w1063:bool)  [unwired: 1 in]
        n444 = case shown="True" w1063 {
          tunnel: w1065 -> [w1067 w1072]
          tunnel: w1064 -> [w1066 w1071]
          tunnel: w1062 -> [_ w1070]
          frame False {
            n445 = Flush Queue(queue=w1067, error in (no error)=w1066) -> ()  [unwired: 3 out]
          }
          frame True {
            n446 = Bundle(cluster=w1070, "state"=state."cam_cnt_acq") -> (w1069:cluster{"state":T4, "value":variant})  [unwired: 1 in]
            n447 = Enqueue Element(queue=w1072, element=w1069, error in (no error)=w1071) -> ()  [unwired: 1 in, 3 out]
          }
        }
      }
      event "center cursor": Value Change {
        n448 = event-data() -> ()  [unwired: 1 in, 6 out]
        n449 = property on="main graph" class="XYGraph (strict)"("Cursor.Cursor X"=500.0 ("Cursor.Cursor Position:Cursor X")) -> ()  [unwired: 2 in, 2 out]
      }
      event "camera max scale": Value Change {
        n450 = event-data() -> ("NewVal"=w1074:u16)  [unwired: 1 in]
        n451 = case shown="2" w1074 {
          tunnel: [65.535 16.384 4.096] -> w1075
          frame 0, Default {
          }
          frame 1 {
          }
          frame 2 {
          }
        }
        n452 = property on="ampl" class="Slide (strict)"("Scale.Maximum"=w1075) -> ()  [unwired: 2 in, 2 out]
      }
      event "ampl": Value Change {
        w1080 = 1000.0 ("y")
        n453 = event-data() -> ()  [unwired: 1 in, 6 out]
        n454 = Unbundle("ampl") -> (w1082:dbl, w1084:dbl)
        n455 = Multiply(x=w1082, y=w1080) -> (x*y=w1081:dbl)
        n456 = Multiply(x=w1084, y=w1080) -> (x*y=w1083:dbl)
        n457 = Max & Min(x=w1081, y=w1083) -> (max(x,y)=w1086:dbl, min(x,y)=w1085:dbl)
        n458 = property on="main graph" class="XYGraph (strict)"("ActYScl"=0 ("Active Y Scale"), "YScale.Maximum"=w1086, "YScale.Minimum"=w1085) -> ()  [unwired: 2 in, 2 out]
      }
      event "Scale.Range:Maximum": Value Change {
        n459 = event-data() -> ("NewVal"=w1088:dbl)  [unwired: 1 in, 5 out]
        n460 = property on="diff" class="Slide (strict)"("Scale.Maximum"=w1088) -> ()  [unwired: 2 in, 2 out]
      }
      event "save wl calibration to .ini": Value Change {
        n461 = event-data() -> ("OldVal"=w1094:bool)  [unwired: 1 in]
        n462 = Bundle(cluster=w1089, "state"=state."dat_save_wl_to_ini") -> (w1093:cluster{"state":T4, "value":variant})  [unwired: 1 in]
        n463 = Enqueue Element(queue=w1090, element=w1093, error in (no error)=w1091) -> ()  [unwired: 1 in, 3 out]
        n464 = property on="save wl calibration to .ini" class="Bool (strict)"("Value"=w1094) -> ()  [unwired: 2 in, 2 out]
      }
      event "stage position(s)": Value Change {
        # "find out which stage is moving"
        n465 = event-data() -> ("NewVal"=w1102:dbl[], "OldVal"=w1105:dbl[])  [unwired: 1 in]
        n466 = for {
          tunnel: w1102 -> [w1110] mode=indexing
          tunnel: w1105 -> [w1108]
          tunnel: [w1109] -> w1101 mode=indexing
          i -> [w1107]
          n467 = Index Array(array=w1108, index=w1107) -> (element=w1106:dbl)
          n468 = Not Equal?(x=w1110, y=w1106) -> (x != y?=w1109:bool)
        }
        n469 = Search 1D Array(1D array=w1101, element=TRUE) -> (index of element=w1097:i32)  [unwired: 1 in]
        "index of element" <- w1097
        n470 = To Variant(anything=w1097) -> (Variant=w1095:variant)
        n471 = Bundle(cluster=w1099, "state"=state."stg_set_pos", "value"=w1095) -> (w1098:cluster{"state":T4, "value":variant})
        n472 = Enqueue Element(queue=w1104, element=w1098, error in (no error)=w1103) -> ()  [unwired: 1 in, 3 out]
      }
      event "set as t0": Value Change {
        n473 = event-data() -> ("NewVal"=w1119:bool[], "OldVal"=w1111:bool[])  [unwired: 1 in]
        n474 = for {
          tunnel: w1119 -> [w1124] mode=indexing
          tunnel: w1111 -> [w1122]
          tunnel: [w1123] -> w1118 mode=indexing
          i -> [w1121]
          n475 = Index Array(array=w1122, index=w1121) -> (element=w1120:bool)
          n476 = Not Equal?(x=w1124, y=w1120) -> (x != y?=w1123:bool)
        }
        n477 = property on="stage position(s)" class="Arr (strict)"() -> ("Value"=w1114:dbl[])  [unwired: 2 in, 2 out]
        n478 = local write "set as t0"(w1111) -> ()
        n479 = Search 1D Array(1D array=w1118, element=TRUE) -> (index of element=w1113:i32)  [unwired: 1 in]
        n480 = Index Array(array=w1114, index=w1113) -> (element=w1112:dbl)
        n481 = Replace Array Subset(array="t0 position(s)", new element=w1112, index=w1113) -> (w1116:dbl[])
        n482 = property on="t0 position(s)" class="Arr (strict)"("Value"=w1116) -> ()  [unwired: 2 in, 2 out]
      }
      event "t0 position(s)": Value Change {
        n483 = event-data() -> ()  [unwired: 1 in, 6 out]
      }
      event "home stages": Value Change {
        # "find out which stage to home"
        n484 = event-data() -> ("NewVal"=w1127:bool[], "OldVal"=w1126:bool[])  [unwired: 1 in]
        n485 = for {
          tunnel: w1127 -> [w1139] mode=indexing
          tunnel: w1126 -> [w1137]
          tunnel: [w1138] -> w1134 mode=indexing
          i -> [w1136]
          n486 = Index Array(array=w1137, index=w1136) -> (element=w1135:bool)
          n487 = Not Equal?(x=w1139, y=w1135) -> (x != y?=w1138:bool)
        }
        n488 = Search 1D Array(1D array=w1134, element=TRUE) -> (index of element=w1131:i32)  [unwired: 1 in]
        n489 = Bundle(cluster=w1130, "state"=state."stg_home", "value"=w1131) -> (w1132:cluster{"state":T4, "value":variant})
        n490 = Enqueue Element(queue=w1129, element=w1132, error in (no error)=w1128) -> ()  [unwired: 1 in, 3 out]
      }
      event "time delay file": Value Change {
        n491 = event-data() -> ("NewVal"=w1141:path)  [unwired: 1 in]
        n492 = To Variant(anything=w1141) -> (Variant=w1140:variant)
        n493 = Bundle(cluster=w1142, "state"=state."scn_load_step_file", "value"=w1140) -> (w1146:cluster{"state":T4, "value":variant})
        n494 = Enqueue Element(queue=w1144, element=w1146, error in (no error)=w1143) -> ()  [unwired: 1 in, 3 out]
      }
      event "scan": Value Change {
        n495 = event-data() -> ("NewVal"=w1147:bool)  [unwired: 1 in]
        n496 = case shown="False" w1147 {
          tunnel: w1150 -> [w1152 w1159]
          tunnel: w1149 -> [w1151 w1158]
          tunnel: w1148 -> [_ w1157]
          frame False {
            n497 = Flush Queue(queue=w1152, error in (no error)=w1151) -> ()  [unwired: 3 out]
          }
          frame True {
            w1155 = 0
            n498 = Build Array(w1155, w1155) -> (w1154:i32[])
            n499 = To Variant(anything=w1154) -> (Variant=w1153:variant)
            n500 = Bundle(cluster=w1157, "state"=state."scn_init", "value"=w1153) -> (w1160:cluster{"state":T4, "value":variant})
            n501 = Enqueue Element(queue=w1159, element=w1160, error in (no error)=w1158) -> ()  [unwired: 1 in, 3 out]
          }
        }
      }
      event "save type": Value Change {
        n502 = event-data() -> ("NewVal"=w1161:bool[])  [unwired: 1 in]
        n503 = To Variant(anything=w1161) -> (Variant=w1163:variant)
        n504 = Bundle(cluster=w1166, "state"=state."dat_update_save_type", "value"=w1163) -> (w1167:cluster{"state":T4, "value":variant})
        n505 = Enqueue Element(queue=w1165, element=w1167, error in (no error)=w1164) -> ()  [unwired: 1 in, 3 out]
      }
      event "index": Value Change {
        n506 = event-data() -> ()  [unwired: 1 in, 2 out]
        n507 = Build Array("index") -> (w1168:u16[])
        n508 = property on="pixel/index" class="Arr (strict)"("Index Values"=w1168) -> ()  [unwired: 2 in, 2 out]
        n509 = property on="wavelength \n(calibration value)" class="Arr (strict)"("Index Values"=w1168) -> ()  [unwired: 2 in, 2 out]
        n510 = property on="wavelength (fitted)" class="Arr (strict)"("Index Values"=w1168) -> ()  [unwired: 2 in, 2 out]
      }
      event "save raw data": Value Change {
        n511 = event-data() -> ("OldVal"=w1175:bool)  [unwired: 1 in]
        n512 = Bundle(cluster=w1171, "state"=state."dat_save_raw") -> (w1170:cluster{"state":T4, "value":variant})  [unwired: 1 in]
        n513 = property on="save raw data" class="Bool (strict)"("Value"=w1175) -> ()  [unwired: 2 in, 2 out]
        n514 = Enqueue Element(queue=w1174, element=w1170, error in (no error)=w1173) -> ()  [unwired: 1 in, 3 out]
      }
      event "save flag": Value Change {
        n515 = event-data() -> ("NewVal"=w1177:bool)  [unwired: 1 in]
        n516 = To Variant(anything=w1177) -> (Variant=w1181:variant)
        n517 = Bundle(cluster=w1180, "state"=state."dat_update_save_flag", "value"=w1181) -> (w1182:cluster{"state":T4, "value":variant})
        n518 = Enqueue Element(queue=w1179, element=w1182, error in (no error)=w1178) -> ()  [unwired: 1 in, 3 out]
      }
      event "view error anal": Value Change {
        n519 = event-data() -> ("NewVal"=w1184:bool)  [unwired: 1 in]
        n520 = vi-ref "error_anal.vi"() -> (w1183:refnum<vi>)
        n521 = case shown="False" w1184 {
          tunnel: w1183 -> [w1189 w1192]
          tunnel: [w1187 w1191] -> w1185
          tunnel: [w1188 w1190] -> w1186
          frame False {
            n522 = invoke class="VI" method="FP.Close"(reference=w1189) -> (reference out=w1188:refnum<vi>, error out=w1187:errorcluster)  [unwired: 2 in, 1 out]
          }
          frame True {
            n523 = invoke class="VI" method="FP.Open"(reference=w1192) -> (reference out=w1190:refnum<vi>, error out=w1191:errorcluster)  [unwired: 4 in, 3 out]
          }
        }
        n524 = Close Reference(reference=w1186, error in (no error)=w1185) -> ()  [unwired: 1 out]
      }
      event "view full data": Value Change {
        n525 = event-data() -> ("NewVal"=w1196:bool)  [unwired: 1 in]
        n526 = vi-ref "view_full_data.vi"() -> (w1195:refnum<vi>)
        n527 = case shown="True" w1196 {
          tunnel: w1195 -> [w1199 w1202]
          tunnel: [w1197 w1201] -> w1193
          tunnel: [w1198 w1200] -> w1194
          frame False {
            n528 = invoke class="VI" method="FP.Close"(reference=w1199) -> (reference out=w1198:refnum<vi>, error out=w1197:errorcluster)  [unwired: 2 in, 1 out]
          }
          frame True {
            n529 = invoke class="VI" method="FP.Open"(reference=w1202) -> (reference out=w1200:refnum<vi>, error out=w1201:errorcluster)  [unwired: 4 in, 3 out]
          }
        }
        n530 = Close Reference(reference=w1194, error in (no error)=w1193) -> ()  [unwired: 1 out]
      }
      event Key Down {
        n531 = event-data() -> ("Char"=w1204:i16)  [unwired: 1 in, 9 out]
        "Char" <- w1204
        n532 = disable-structure shown="Disabled" {
          disable-tunnel: w1204 -> [w1205 _]
          frame Disabled {
            n533 = case shown="49" w1205 {
              frame 0, Default {
              }
              frame 49 {
                n534 = property on="stage position(s)" class="Arr (strict)"("Array Element.Key Focus"=TRUE) -> ()  [unwired: 2 in, 2 out]
              }
              frame 98 {
                n535 = property on="get bg" class="Bool (strict)"() -> ("Value"=w1208:bool)  [unwired: 2 in, 2 out]
                n536 = Not(x=w1208) -> (.not. x?=w1207:bool)
                n537 = property on="get bg" class="Bool (strict)"("Val(Sgnl)"=w1207) -> ()  [unwired: 2 in, 2 out]
              }
              frame 99 {
                n538 = property on="cont acq" class="Bool (strict)"() -> ("Value"=w1210:bool)  [unwired: 2 in, 2 out]
                n539 = Not(x=w1210) -> (.not. x?=w1209:bool)
                n540 = property on="cont acq" class="Bool (strict)"("Val(Sgnl)"=w1209) -> ()  [unwired: 2 in, 2 out]
              }
              frame 115 {
                n541 = property on="get_single_acq" class="Bool (strict)"("Val(Sgnl)"=TRUE ("Value (Signaling)")) -> ()  [unwired: 2 in, 2 out]
              }
            }
          }
          frame Enabled {
          }
        }
        n542 = Wait (ms)(milliseconds to wait=u32 75) -> ()  [unwired: 1 out]
      }
      event Panel Close? {
        w1217 = TRUE
        n543 = event-data() -> ()  [unwired: 1 in, 4 out]
        n544 = Bundle(cluster=w1214, "state"=state."stop" ("element")) -> (w1212:cluster{"state":T4, "value":variant})  [unwired: 1 in]
        n545 = Enqueue Element(queue=w1216, element=w1212, error in (no error)=w1215) -> ()  [unwired: 1 in, 3 out]
        n546 = event-data("Discard?"=w1217) -> ()  [unwired: 1 in, 1 out]
      }
    }
  }
  n547 = call <vilib>:"Simple Error Handler.vi"("error in (no error)"=w71) -> ()  [unwired: 4 in, 5 out]
